vi "Main.vi"(8 "error in":errorcluster, 11 "UI SmarAct in":refnum<class "UI SmarAct.lvclass">) -> (0 "error out":errorcluster, 3 "UI SmarAct out":refnum<class "UI SmarAct.lvclass">)   [LabVIEW 2024, in "UI SmarAct.lvclass"]
doc: "The <b>Queued Message Handler</b> of the Worker that owns this VI."
uses:
  UI SmarAct.lvclass
  C:/Program Files (x86)/National Instruments/LabVIEW 2024/vi.lib/addons/_Workers/Library/Classes/Worker/Worker.lvclass
  <vilib>/addons/_Workers/Library/Classes/Message Queue/Message Queue.lvclass
  <vilib>/addons/_Workers/Library/Classes/Error Handler/Error Handler.lvclass
  <vilib>/addons/_Workers/Library/Classes/Message/Message.lvclass
  <vilib>/addons/_Workers/Library/Classes/EHL/EHL.lvclass
  <vilib>/addons/_Workers/Library/Classes/Workers Object/Workers Object.lvclass
  Spectro Acquisition/Spectro Acquisition.lvclass
  File manipulate/File manipulate.lvclass
  Initialization Data.ctl
  Response Cases.ctl
  UI SmarAct.lvclass/UI SmarAct.ctl
  rql_Connect MCS.ctl
  rql_Update channel.ctl
  rql_Update Vitesse.ctl
  rql_Switch Platine.ctl
  rql_Update Port COM.ctl
  rql_Update Tps Int.ctl
  Spectro Acquisition/rqp_Appliquer BKG.ctl
  rql_Update Calib.ctl
  rql_Update Incr Scan.ctl
  rql_Update fin scan.ctl
  rql_Save Spectrogramme.ctl
  rql_Update Pas Platine.ctl
  rql_Update Controller Adress SMC100.ctl
  Status Platine.ctl
  rql_Refresh.ctl
  rql_Write init file.ctl
  rql_Get position.ctl
  rql_Set Zero Position.ctl
  rql_Find Reference Zero.ctl
  rql_Forward CloseLoop.ctl
  rql_Stop platine.ctl
  rql_Status Position Platine.ctl
  Spectro Acquisition/rqp_Set Int Time.ctl
  rql_Start Acquisition.ctl
  Spectro Acquisition/rqp_Start Acquisition.ctl
  rql_Start Scan.ctl
  File manipulate/rqp_Save Spectrogramme Data.ctl
  Spectro Acquisition/rqp_Appliquer calibration.ctl
  fed1715e-ad66-47da-94cb-5b802a3bcd4b.vi
  338c79d3-4f60-42bd-8753-b5f43bf2242e.vi
  b1e2cd65-b1f1-482f-a644-3403d26b6092.vi
  193bb31d-fb75-400f-a6aa-d82127e562de.vi
  cd9d0536-fc44-4fa3-b225-ca8b7675d591.vi
  9cd4564f-d818-4b39-8ead-d47f8c0a47b5.vi
  <vilib>/ErrorRing/Error Ring.xnode
  <vilib>/addons/_Workers/Debugger/Debug Client/Debug Client.lvlib
panel:
  in  "Commande onglets":T1(tab)
  out "Status Platine":bool
  in  "Platine Newport":enum32{"Initialisation", "Commandes"}(tab)
  in  "Port COM":refnum<visa-resource-name>
  in  "Adresse SMC100":i32
  out "Version Controller":string
  in  "Inc Scan:(um)":dbl step=0.001 format="%#_6f"
  out "fs 3":ext caption="fs" format="%.2f fs"
  out "fs2":ext caption="fs" format="%.2f fs"
  in  "Stop Scan":bool
  in  "fin (um)":i32
  in  "Début (um)":i32
  in  "Start Scan":bool
  out "scan en cours(N)":i32
  in  "Calib?":bool caption="Checkbox"
  in  "BKG":bool
  in  "Stop Acquisition":bool
  in  "Start Acquisition":bool
  in  "Tps Int.(ms)":u32
  out "Connect Spectro?":bool
  in  "Connecter Spectro":bool
  out "Spectrometer Name":string
  out "Serial Number":string
  in  "BKG?":bool caption="Checkbox"
  in  "Platine Switch":bool
  out "Modèle platine":string
  out "fs":ext format="%.2f"
  in  "speed (0 ... 100 000 000)":u32=1000000 max=100000000 step=1
  in  "Channel":u32
  in  "get position":bool
  out "um":dbl format="%.2f"
  in  "Set Zero":bool
  in  "Find Zero":bool
  in  "max freq (50 ... 18 500)":u32=200 min=50 max=18500 step=1
  in  "Stop moteur":bool
  in  "Abs/Rel":bool caption="Checkbox"
  in  "Back CL":bool
  in  "Forward CL":bool
  in  "Inc:(um)":dbl step=0.001 format="%#_6f"
  out "Connect?":bool
  in  "Connecter":bool
  in  "Select MCS":u16(ring)
  in  "Refresh":bool
  out "FWHM(Gauss)":dbl
  out "FWHM(Sech2)":dbl
  out "Aire":dbl
  out "Transposer Le spectrogramme":bool
  in  "Save FROG Trace":bool
  out "Zoom Spectre":cluster{dbl[], dbl[]}(graph)
  out "PosX.Curs-1":dbl
  out "PosX.Curs-0":dbl
  out "Spectre":T2(graph)
  out "Autoccorrélation":dbl[][](graph)
  out "FROG Trace":dbl[][](graph)
  # "Commande Platine Newport"
  # "Scan Platine-Spectro"
  # "Commande Spectromètre"
  # "Modèle Platine :"
  # "Commande Platine MCS"
  # "Commande Platine Closed-Loop"
  # "Connection MCS"
  # "Autoccorrélation"
  # "Reconstruction"
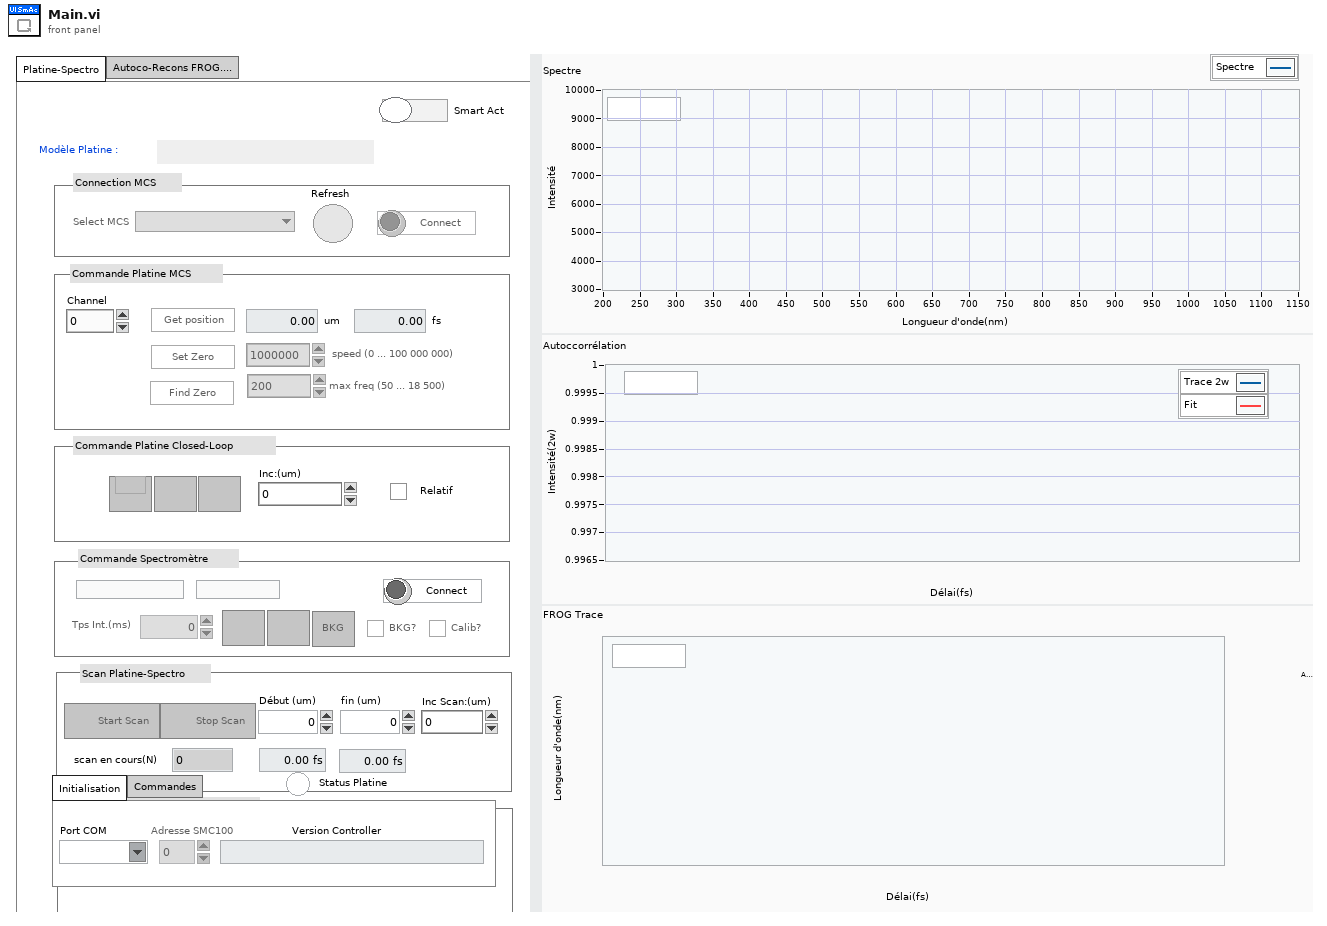
[diagram p1: front panel]
types:
  T1 = enum32{"Platine-Spectro", "Autoco-Recons FROG...."}
  T2 = cluster{"Spectre-BKG":dbl[], "Wavelenghts":dbl[]}
  T3 = cluster{"Wavelenghts":dbl[], "Spectre-BKG":dbl[]}
  T4 = typedef "UI SmarAct.lvclass/Initialization Data.ctl" = cluster{"Response Cases":T5}
  T5 = typedef "UI SmarAct.lvclass/Response Cases.ctl" = cluster{"Placeholder - Can be deleted":string, "Channel":u32, "chemin fichier init":path, "max freq (50 ... 18 500)":u32, "speed (0 ... 100 000 000)":u32, "Abs/Rel":bool, "Tps Int(ms)":u32, "Modèle Platine":string, "Début (um)":i32, "fin (um)":i32, "Inc:(um)":dbl, "Platine Switch":bool, "Port COM":refnum<visa-resource-name>, "Calib?":bool, "Inc Scan:(um)":dbl, "Adresse SMC100":i32}
  T6 = typedef "UI SmarAct.lvclass/Status Platine.ctl" = enum16{"En mouvement...", "Stopée", "Veille"}
  T7 = typedef "UI SmarAct.lvclass/rql_Connect MCS.ctl" = cluster{"String":string, "Connect?":bool}
  T8 = typedef "UI SmarAct.lvclass/rql_Refresh.ctl" = cluster{"String":string}
  T9 = typedef "UI SmarAct.lvclass/rql_Write init file.ctl" = cluster{"String":string}
  T10 = typedef "UI SmarAct.lvclass/rql_Update channel.ctl" = cluster{"Channel":u32}
  T11 = enum32{"SA_SENSOR_DISABLED", "SA_SENSOR_ENABLED", "SA_SENSOR_POWERSAVE"}
  T12 = typedef "UI SmarAct.lvclass/rql_Get position.ctl" = cluster{"String":string}
  T13 = typedef "UI SmarAct.lvclass/rql_Set Zero Position.ctl" = cluster{"String":string}
  T14 = enum32{"SA_FORWARD_DIRECTION", "SA_BACKWARD_DIRECTION", "SA_FORWARD_BACKWARD_DIRECTION", "SA_BACKWARD_FORWARD_DIRECTION", "SA_FORWARD_DIRECTION_ABORT_ON_ENDSTOP", "SA_BACKWARD_DIRECTION_ABORT_ON_ENDSTOP", "SA_FORWARD_BACKWARD_DIRECTION_ABORT_ON_ENDSTOP", "SA_BACKWARD_FORWARD_DIRECTION_ABORT_ON_ENDSTOP"}
  T15 = typedef "UI SmarAct.lvclass/rql_Find Reference Zero.ctl" = cluster{"String":string}
  T16 = typedef "UI SmarAct.lvclass/rql_Forward CloseLoop.ctl" = cluster{"String":string}
  T17 = typedef "UI SmarAct.lvclass/rql_Update Fréquence.ctl" = cluster{"max freq (50 ... 18 500)":u32}
  T18 = typedef "UI SmarAct.lvclass/rql_Update Vitesse.ctl" = cluster{"speed (0 ... 100 000 000)":u32}
  T19 = typedef "UI SmarAct.lvclass/rql_Mode déplacement.ctl" = cluster{"Abs/Rel":bool}
  T20 = typedef "UI SmarAct.lvclass/rql_Initialise Spectromètre.ctl" = cluster{"Connecter Spectro?":bool}
  T21 = typedef "UI SmarAct.lvclass/rql_Stop platine.ctl" = cluster{"String":string}
  T22 = typedef "UI SmarAct.lvclass/rql_Status Position Platine.ctl" = cluster{"String":string}
  T23 = typedef "Spectro Acquisition.lvclass/rqp_Set Int Time.ctl" = cluster{"Tps Int(ms)":u32}
  T24 = typedef "UI SmarAct.lvclass/rql_Update Tps Int.ctl" = cluster{"Tps Int.(ms)":u32}
  T25 = typedef "Spectro Acquisition.lvclass/rqp_Start Acquisition.ctl" = cluster{"Wrapper Spectro":u32}
  T26 = typedef "UI SmarAct.lvclass/rql_Start Acquisition.ctl" = cluster{"String":string}
  T27 = typedef "UI SmarAct.lvclass/rql_Start Scan.ctl" = cluster{"String":string}
  T28 = typedef "UI SmarAct.lvclass/rql_Update début scan.ctl" = cluster{"Début (um)":i32}
  T29 = typedef "UI SmarAct.lvclass/rql_Update fin scan.ctl" = cluster{"fin (um)":i32}
  T30 = typedef "File manipulate.lvclass/rqp_Save Spectrogramme Data.ctl" = cluster{"Save SpecTG":bool, "Paramètres longueur d'onde":T31, "FROG Trace":dbl[][], "pas (um)":dbl, "Nbre de scans":i32, "WL Values":dbl[], "Transposer L'image":bool}
  T31 = typedef "UI SmarAct.lvclass/Paramètres longueur d'onde.ctl" = cluster{"N":i32, "lambda_0":dbl, "lambda_c":dbl, "d_lambda":dbl}
  T32 = typedef "UI SmarAct.lvclass/rql_Save Spectrogramme.ctl" = cluster{"Save":bool}
  T33 = typedef "UI SmarAct.lvclass/rql_Update Pas Platine.ctl" = cluster{"Inc:(um)":dbl}
  T34 = typedef "UI SmarAct.lvclass/rql_Switch Platine.ctl" = cluster{"Platine Switch":bool}
  T35 = typedef "UI SmarAct.lvclass/rql_Update Port COM.ctl" = cluster{"Port COM":refnum<visa-resource-name>}
  T36 = typedef "Spectro Acquisition.lvclass/rqp_Appliquer calibration.ctl" = cluster{"Calib?":bool}
  T37 = typedef "UI SmarAct.lvclass/rql_Update Calib.ctl" = cluster{"Calib?":bool}
  T38 = typedef "UI SmarAct.lvclass/rql_Update Incr Scan.ctl" = cluster{"Inc Scan:(um)":dbl}
  T39 = typedef "UI SmarAct.lvclass/rql_Update Controller Adress SMC100.ctl" = cluster{"Adresse SMC100":i32}
  T40 = typedef "Spectro Acquisition.lvclass/rqp_Appliquer BKG.ctl" = cluster{"BackGround?":bool}
  T41 = enum32{"SA_STOPPED_STATUS", "SA_STEPPING_STATUS", "SA_SCANNING_STATUS", "SA_HOLDING_STATUS", "SA_TARGET_STATUS", "SA_MOVE_DELAY_STATUS", "SA_CALIBRATING_STATUS", "SA_FINDING_REF_STATUS", "SA_OPENING_STATUS"}
  T42 = enum32{"invalid app kind", "Development System", "Run Time System", "Student Edition", "Embedded LabVIEW", "Evaluation", "Custom"}
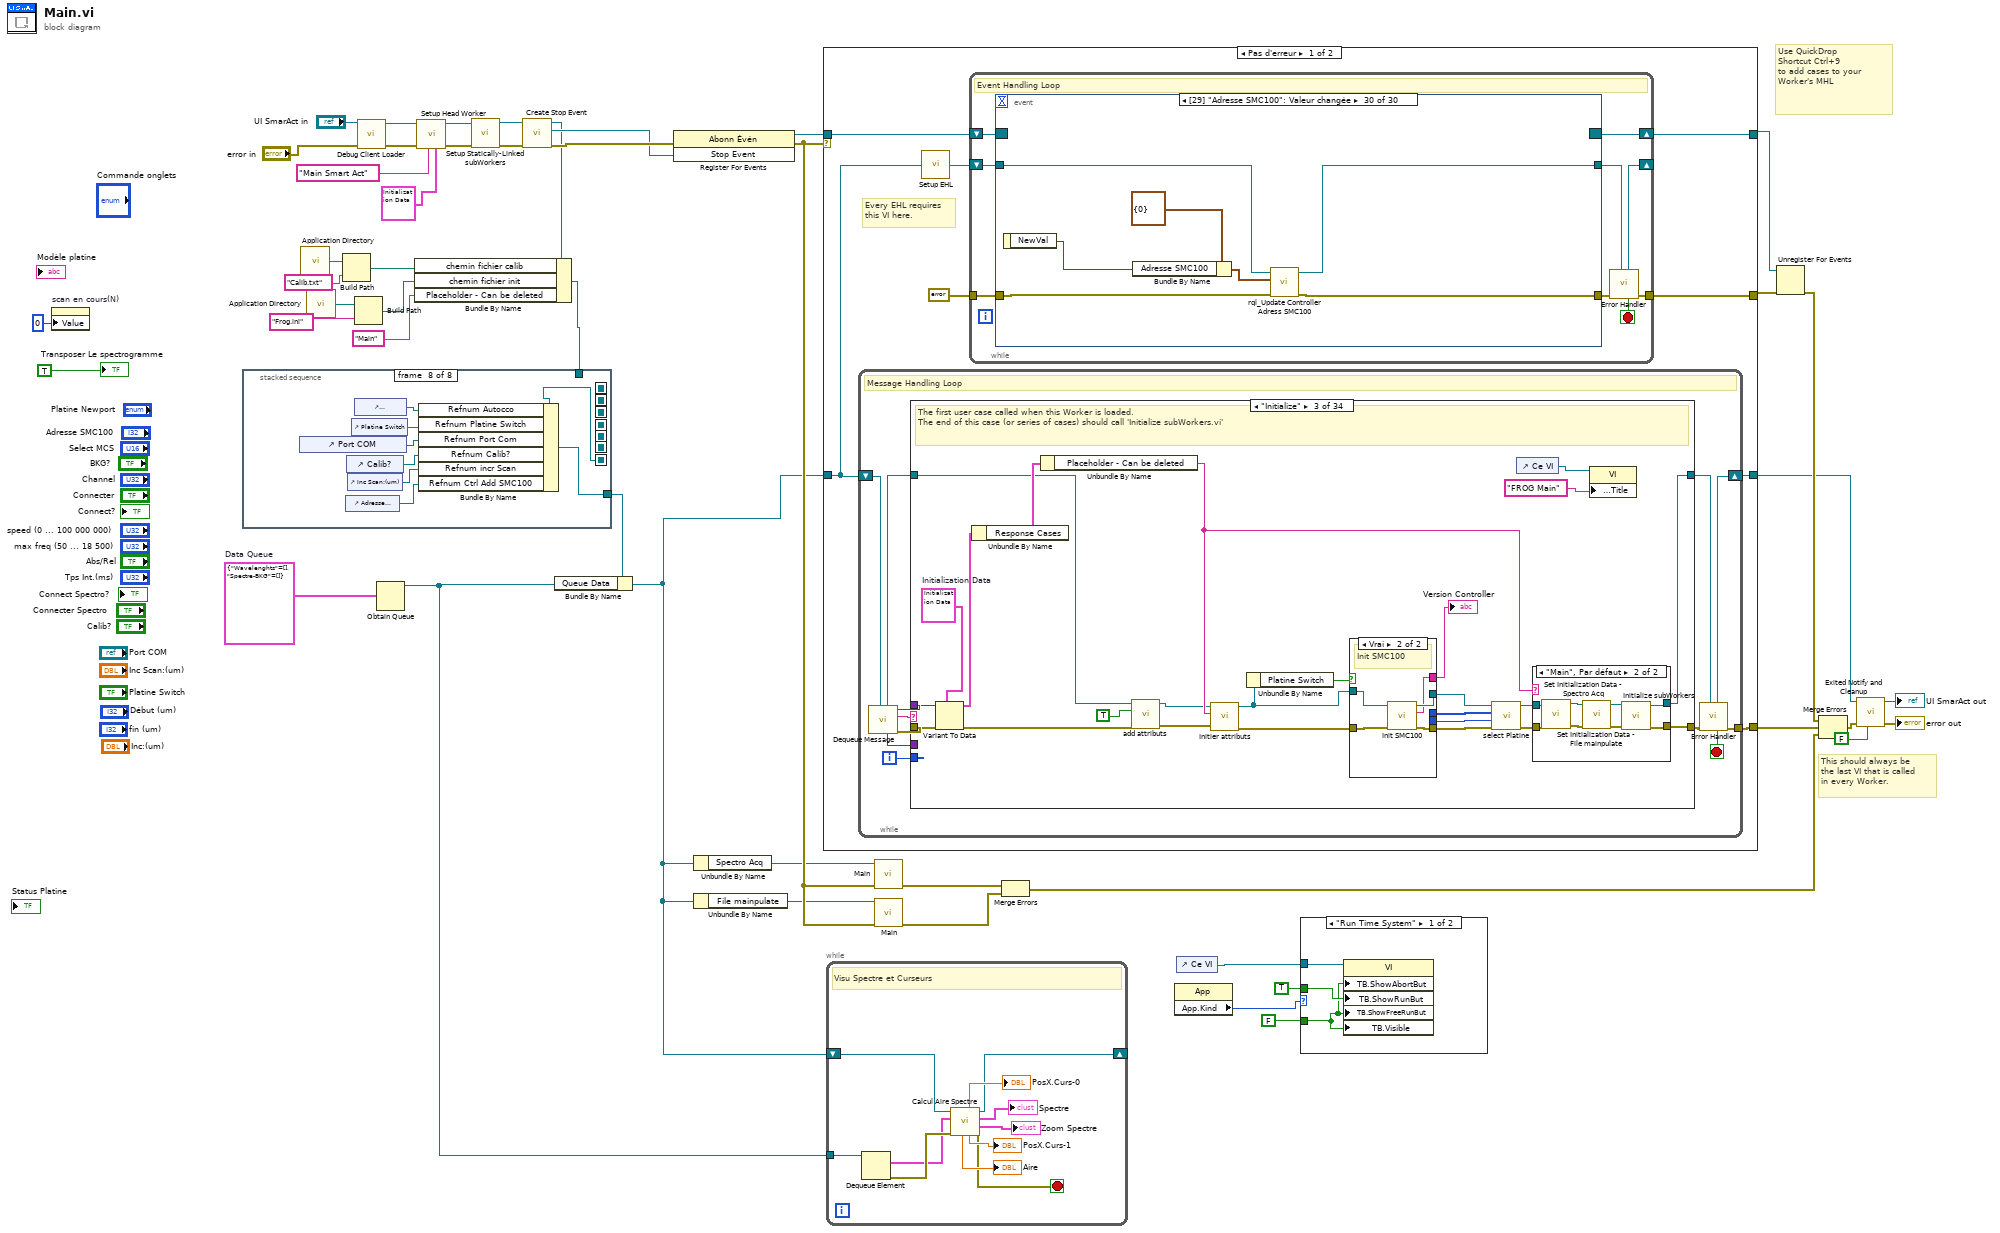
[diagram p0: block diagram]
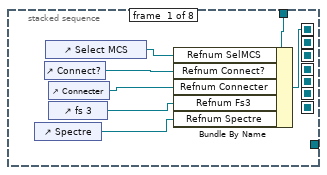
[diagram p2: hidden frame]
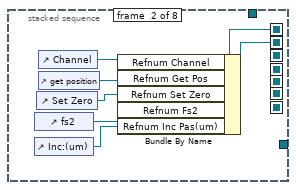
[diagram p3: hidden frame]
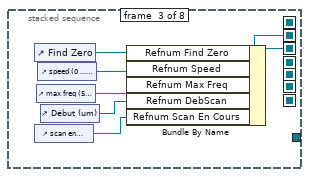
[diagram p4: hidden frame]
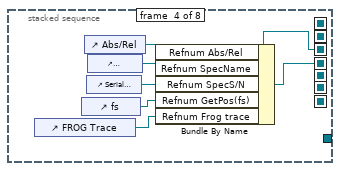
[diagram p5: hidden frame]
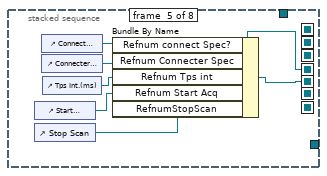
[diagram p6: hidden frame]
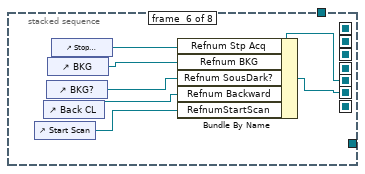
[diagram p7: hidden frame]
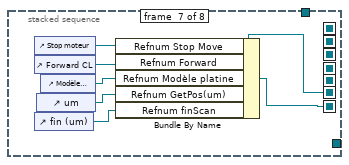
[diagram p8: hidden frame]
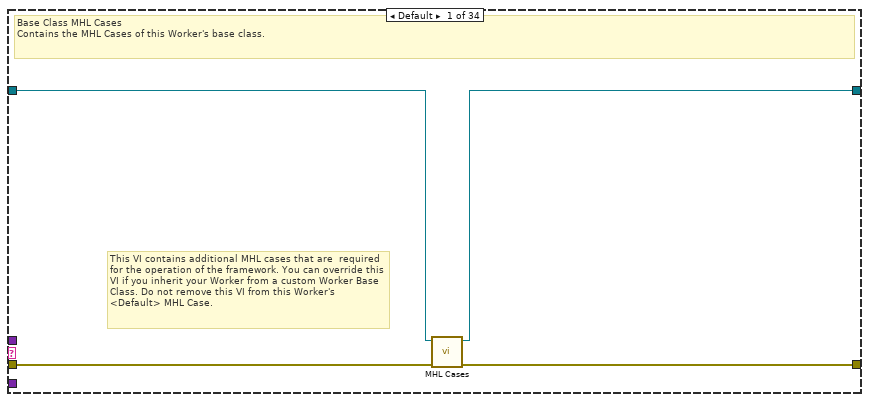
[diagram p10: hidden frame]
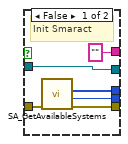
[diagram p12: hidden frame]
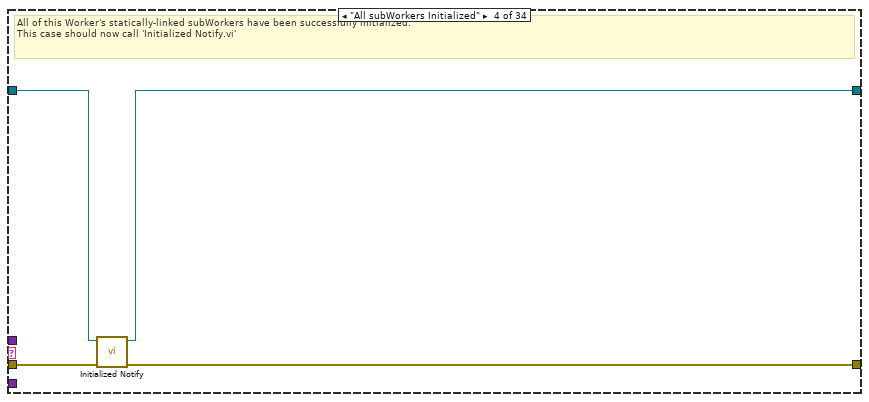
[diagram p14: hidden frame]
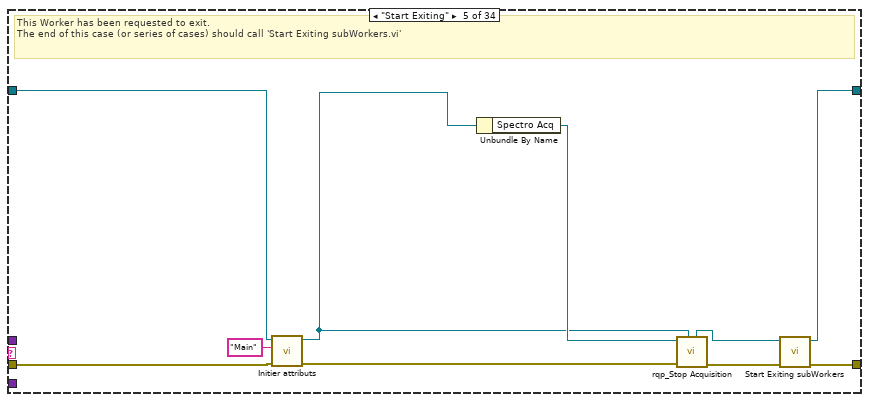
[diagram p15: hidden frame]
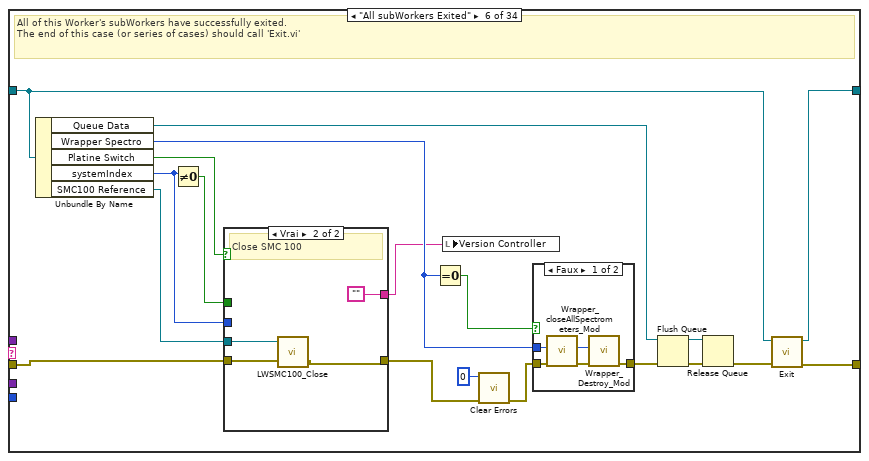
[diagram p16: hidden frame]
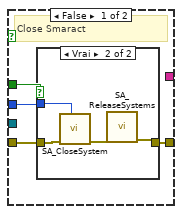
[diagram p17: hidden frame]
diagram:
  w23 = T3 {"Wavelenghts"=[], "Spectre-BKG"=[]}  # Data Queue
  # "Use QuickDrop\nShortcut Ctrl+9\nto add cases to your\nWorker's MHL"
  # "This should always be the last VI that is called in every Worker."
  n1 = property on="scan en cours(N)" class="NumNb (strict)"("Value"=0 ("scan en cours(N)")) -> ()  [unwired: 2 in, 2 out]
  n2 = call <vilib>:"Application Directory.vi"() -> ("Application Directory"=w13:path)
  n3 = call <vilib>:"Application Directory.vi"() -> ("Application Directory"=w33:path)
  n4 = Build Path(base path=w13, name or relative path="Calib.txt") -> (appended path=w7:path)
  n5 = Build Path(base path=w33, name or relative path="Frog.ini") -> (appended path=w6:path)
  n6 = call <vilib>:"Debug Client Loader.vi"("error in (no error)"="error in", "Worker_"="UI SmarAct in") -> ("error out"=w16:errorcluster, "Worker_out"=w15:refnum<class "UI SmarAct.lvclass">)  [unwired: 8 in]
  n7 = Obtain Queue(element data type=w23) -> (queue out=w3:refnum<queue>)  [unwired: 4 in, 2 out]
  n8 = call-dynamic "Setup Head Worker.vi"("Initalization Data"=T4 {"Response Cases"={"Placeholder - Can be deleted"="", "Channel"=0, "chemin fichier init"=path "", "max freq (50 ... 18 500)"=200, "speed (0 ... 100 000 000)"=1000000, "Abs/Rel"=FALSE, "Tps Int(ms)"=0, "Modèle Platine"="", "Début (um)"=0, "fin (um)"=0, "Inc:(um)"=0.0, "Platine Switch"=FALSE, "Port COM"="", "Calib?"=FALSE, "Inc Scan:(um)"=0.0, "Adresse SMC100"=0}} ("Initialization Data"), "Worker Alias"="Main Smart Act", "error in"=w16, "Worker_"=w15) -> ("error out"=w24:errorcluster, "Worker_out"=w27:refnum<class "UI SmarAct.lvclass">)  [unwired: 6 in]
  n9 = call "Setup Statically-Linked subWorkers.vi"("error in"=w24, "UI SmarAct in"=w27) -> ("error out"=w25:errorcluster, "UI SmarAct out"=w26:refnum<class "UI SmarAct.lvclass">)  [unwired: 8 in]
  n10 = call-dynamic "Create Stop Event.vi"("error in"=w25, "Worker"=w26) -> ("error out"=w42:errorcluster, "Stop Event"=w39:refnum<user-event>, "Worker out"=w8:refnum<class "UI SmarAct.lvclass">)  [unwired: 7 in]
  n11 = Bundle By Name ("Assembler par nom")(cluster=w8, "chemin fichier calib"=w7, "chemin fichier init"=w6, "Placeholder - Can be deleted"="Main" ("Response Cases.Placeholder - Can be deleted")) -> (w2:refnum<class "UI SmarAct.lvclass">)
  n12 = stacked-sequence {
    seq-local: [w51 _ _ _ _ _ _ _] -> [_ w61 _ _ _ _ _ _]
    seq-local: [_ w60 _ _ _ _ _ _] -> [_ _ w68 _ _ _ _ _]
    seq-local: [_ _ w64 _ _ _ _ _] -> [_ _ _ w75 _ _ _ _]
    seq-local: [_ _ _ w71 _ _ _ _] -> [_ _ _ _ w78 _ _ _]
    seq-local: [_ _ _ _ w77 _ _ _] -> [_ _ _ _ _ w85 _ _]
    seq-local: [_ _ _ _ _ w84 _ _] -> [_ _ _ _ _ _ w92 _]
    seq-local: [_ _ _ _ _ _ w90 _] -> [_ _ _ _ _ _ _ w98]
    tunnel: w2 -> [w52 _ _ _ _ _ _ _]
    tunnel: [_ _ _ _ _ _ _ w99] -> w1
    frame #0 {
      n13 = control-ref of="Spectre"() -> (w48:refnum<vi>)
      n14 = control-ref of="Connect?"() -> (w53:refnum<vi>)
      n15 = control-ref of="Select MCS"() -> (w54:refnum<vi>)
      n16 = control-ref of="Connecter"() -> (w50:refnum<vi>)
      n17 = control-ref of="fs 3"() -> (w49:refnum<vi>)
      n18 = Bundle By Name ("Assembler par nom")(cluster=w52, "Refnum SelMCS"=w54, "Refnum Connect?"=w53, "Refnum Connecter"=w50, "Refnum Fs3"=w49, "Refnum Spectre"=w48) -> (w51:refnum<class "UI SmarAct.lvclass">)
    }
    frame #1 {
      n19 = control-ref of="fs2"() -> (w56:refnum<vi>)
      n20 = control-ref of="Inc:(um)"() -> (w55:refnum<vi>)
      n21 = control-ref of="Set Zero"() -> (w57:refnum<vi>)
      n22 = control-ref of="Channel"() -> (w59:refnum<vi>)
      n23 = control-ref of="get position"() -> (w58:refnum<vi>)
      n24 = Bundle By Name ("Assembler par nom")(cluster=w61, "Refnum Channel"=w59, "Refnum Get Pos"=w58, "Refnum Set Zero"=w57, "Refnum Fs2"=w56, "Refnum Inc Pas(um)"=w55) -> (w60:refnum<class "UI SmarAct.lvclass">)
    }
    frame #2 {
      n25 = control-ref of="Find Zero"() -> (w65:refnum<vi>)
      n26 = control-ref of="scan en cours(N)"() -> (w62:refnum<vi>)
      n27 = control-ref of="max freq (50 ... 18 500)"() -> (w67:refnum<vi>)
      n28 = control-ref of="speed (0 ... 100 000 000)"() -> (w66:refnum<vi>)
      n29 = control-ref of="Début (um)"() -> (w63:refnum<vi>)
      n30 = Bundle By Name ("Assembler par nom")(cluster=w68, "Refnum Find Zero"=w65, "Refnum Speed"=w66, "Refnum Max Freq"=w67, "Refnum DebScan"=w63, "Refnum Scan En Cours"=w62) -> (w64:refnum<class "UI SmarAct.lvclass">)
    }
    frame #3 {
      n31 = control-ref of="FROG Trace"() -> (w69:refnum<vi>)
      n32 = control-ref of="fs"() -> (w70:refnum<vi>)
      n33 = control-ref of="Abs/Rel"() -> (w74:refnum<vi>)
      n34 = control-ref of="Serial Number"() -> (w72:refnum<vi>)
      n35 = control-ref of="Spectrometer Name"() -> (w73:refnum<vi>)
      n36 = Bundle By Name ("Assembler par nom")(cluster=w75, "Refnum Abs/Rel"=w74, "Refnum SpecName"=w73, "Refnum SpecS/N"=w72, "Refnum GetPos(fs)"=w70, "Refnum Frog trace"=w69) -> (w71:refnum<class "UI SmarAct.lvclass">)
    }
    frame #4 {
      n37 = control-ref of="Start Acquisition"() -> (w79:refnum<vi>)
      n38 = control-ref of="Stop Scan"() -> (w76:refnum<vi>)
      n39 = control-ref of="Connect Spectro?"() -> (w82:refnum<vi>)
      n40 = control-ref of="Connecter Spectro"() -> (w81:refnum<vi>)
      n41 = control-ref of="Tps Int.(ms)"() -> (w80:refnum<vi>)
      n42 = Bundle By Name ("Assembler par nom")(cluster=w78, "Refnum connect Spec?"=w82, "Refnum Connecter Spec"=w81, "Refnum Tps int"=w80, "Refnum Start Acq"=w79, "RefnumStopScan"=w76) -> (w77:refnum<class "UI SmarAct.lvclass">)
    }
    frame #5 {
      n43 = control-ref of="Start Scan"() -> (w83:refnum<vi>)
      n44 = control-ref of="Back CL"() -> (w86:refnum<vi>)
      n45 = control-ref of="BKG?"() -> (w87:refnum<vi>)
      n46 = control-ref of="BKG"() -> (w88:refnum<vi>)
      n47 = control-ref of="Stop Acquisition"() -> (w89:refnum<vi>)
      n48 = Bundle By Name ("Assembler par nom")(cluster=w85, "Refnum Stp Acq"=w89, "Refnum BKG"=w88, "Refnum SousDark?"=w87, "Refnum Backward"=w86, "RefnumStartScan"=w83) -> (w84:refnum<class "UI SmarAct.lvclass">)
    }
    frame #6 {
      n49 = control-ref of="Stop moteur"() -> (w96:refnum<vi>)
      n50 = control-ref of="Forward CL"() -> (w95:refnum<vi>)
      n51 = control-ref of="fin (um)"() -> (w91:refnum<vi>)
      n52 = control-ref of="um"() -> (w93:refnum<vi>)
      n53 = control-ref of="Modèle platine"() -> (w94:refnum<vi>)
      n54 = Bundle By Name ("Assembler par nom")(cluster=w92, "Refnum Stop Move"=w96, "Refnum Forward"=w95, "Refnum Modèle platine"=w94, "Refnum GetPos(um)"=w93, "Refnum finScan"=w91) -> (w90:refnum<class "UI SmarAct.lvclass">)
    }
    frame #7 {
      n55 = control-ref of="Port COM"() -> (w102:refnum<vi>)
      n56 = control-ref of="Adresse SMC100"() -> (w97:refnum<vi>)
      n57 = control-ref of="Calib?"() -> (w101:refnum<vi>)
      n58 = control-ref of="Inc Scan:(um)"() -> (w100:refnum<vi>)
      n59 = control-ref of="Platine Switch"() -> (w103:refnum<vi>)
      n60 = control-ref of="Autoccorrélation"() -> (w104:refnum<vi>)
      n61 = Bundle By Name ("Assembler par nom")(cluster=w98, "Refnum Autocco"=w104, "Refnum Platine Switch"=w103, "Refnum Port Com"=w102, "Refnum Calib?"=w101, "Refnum incr Scan"=w100, "Refnum Ctrl Add SMC100"=w97) -> (w99:refnum<class "UI SmarAct.lvclass">)
    }
  }
  n62 = Bundle By Name ("Assembler par nom")(cluster=w1, "Queue Data"=w3) -> (w4:refnum<class "UI SmarAct.lvclass">)
  n63 = register-events(error in=w42, w39) -> (reference out=w41:refnum<event-registration>, error out=w36:errorcluster)  [unwired: 1 in]
  n64 = Unbundle By Name(w4) -> ("Spectro Acq"=w10:refnum<class "Spectro Acquisition.lvclass">)
  n65 = Unbundle By Name(w4) -> ("File mainpulate"=w9:refnum<class "File manipulate.lvclass">)
  n66 = case shown="Pas d'erreur" w36 {
    tunnel: w4 -> [w107 w942]
    tunnel: [w105 w943] -> w40
    tunnel: w41 -> [w112 w944]
    tunnel: [w109 w945] -> w46
    tunnel: [w111 w944] -> w45
    tunnel: [w106 w941] -> w43
    selector: w36 -> [_ w945]
    frame No Error {
      # "Every EHL requires\nthis VI here."
      n67 = while {
        shift-right: [w122] -> w106
        shift-left: w107 -> [w124]
        tunnel: [w123] -> w105
        i -> [w115]
        stop <- w116 stop-if-true
        # "Message Handling Loop"
        n68 = call-dynamic "Dequeue Message.vi"("Worker"=w124) -> ("error out"=w121:errorcluster, "Case out"=w117:string, "Data out"=w113:variant, "Auxiliary out"=w114:variant, "Worker out"=w119:refnum<class "UI SmarAct.lvclass">)  [unwired: 6 in]
        n69 = case "Worker MHL Case Structure (DO NOT CHANGE LABEL NAME)" shown="\"Initialize\"" w117 {
          tunnel: w121 -> [w128 w129 w155 w178 w187 w206 w230 w247 w270 w279 w288 w312 w324 w336 w354 w402 w442 w453 w464 w478 w492 w505 w551 w563 w574 w639 w652 w672 w682 w696 w710 w728 w740 w753]
          tunnel: [w127 w129 w144 w177 w190 w209 w230 w234 w261 w273 w283 w304 w315 w330 w354 w393 w439 w445 w459 w468 w488 w500 w547 w556 w570 w628 w642 w666 w677 w689 w705 w716 w730 w745] -> w120
          tunnel: w119 -> [w126 w130 w139 w180 w188 w207 w229 w242 w260 w272 w289 w307 w314 w327 w343 w388 w436 w454 w458 w472 w487 w496 w552 w559 w567 w632 w653 w660 w676 w697 w711 w718 w741 w754]
          tunnel: [w125 w130 w143 w179 w189 w208 w229 w233 w265 w271 w281 w307 w313 w327 w345 w385 w438 w443 w457 w465 w486 w498 w546 w559 w569 w626 w645 w664 w675 w688 w704 w714 w732 w743] -> w118
          tunnel: w115 -> [_ _ _ _ _ _ _ _ _ _ _ _ _ _ _ _ _ _ _ _ _ _ _ _ _ _ _ _ _ _ _ _ _ _]
          tunnel: w114 -> [_ _ _ _ _ _ _ _ _ _ _ _ _ _ _ _ _ _ _ _ _ _ _ _ _ _ _ _ _ _ _ _ _ _]
          tunnel: w113 -> [_ _ w154 _ _ _ _ w245 w268 w277 w286 w310 w322 w334 w352 w399 w440 w451 w462 w476 w490 w503 w549 w561 w572 w637 w650 w670 w680 w693 w708 w725 w737 w750]
          frame Default {
            # "This VI contains additional MHL cases that are  required for the operation of the framework. You can override this VI if you inherit your Worker from a custom Worker Base Class. Do not remove this VI from this Worker's <Default> MHL Case."
            # "Base Class MHL Cases\nContains the MHL Cases of this Worker's base class."
            n70 = call-dynamic "MHL Cases.vi"("error in"=w128, "Worker in"=w126) -> ("error out"=w127:errorcluster, "Worker out"=w125:refnum<class "UI SmarAct.lvclass">)  [unwired: 8 in]
          }
          frame "------------ FRAMEWORK CASES -----------" {
            # "Start of Workers Framework Cases"
          }
          frame "Initialize" {
            w153 = T4 {"Response Cases"={"Placeholder - Can be deleted"="", "Channel"=0, "chemin fichier init"=path "", "max freq (50 ... 18 500)"=200, "speed (0 ... 100 000 000)"=1000000, "Abs/Rel"=FALSE, "Tps Int(ms)"=0, "Modèle Platine"="", "Début (um)"=0, "fin (um)"=0, "Inc:(um)"=0.0, "Platine Switch"=FALSE, "Port COM"="", "Calib?"=FALSE, "Inc Scan:(um)"=0.0, "Adresse SMC100"=0}}  # Initialization Data
            # "The first user case called when this Worker is loaded.\nThe end of this case (or series of cases) should call 'Initialize subWorkers.vi'"
            n71 = Variant To Data(error in=w155, type=w153, Variant=w154) -> (data=w148:T4, error out=w137:errorcluster)
            n72 = Unbundle By Name(w148) -> ("Response Cases"=w147:T5)
            n73 = Unbundle By Name(w147) -> ("Placeholder - Can be deleted"=w142:string)
            n74 = call "add attributs.vi"("error in (no error)"=w137, "Read/Write"=TRUE, "UI SA en entrée"=w139) -> ("error out"=w136:errorcluster, "UI SA en sortie"=w138:refnum<class "UI SmarAct.lvclass">)  [unwired: 7 in]
            n75 = call "Initier attributs.vi"("error in (no error)"=w136, "Main/Refresh"=w142, "UI SA en entrée"=w138) -> ("error out"=w149:errorcluster, "UI SA en sortie"=w133:refnum<class "UI SmarAct.lvclass">)  [unwired: 7 in]
            n76 = Unbundle By Name(w133) -> ("Platine Switch"=w134:bool)
            n77 = case shown="Vrai" w134 {
              tunnel: [w161 _] -> w152
              tunnel: [w160 _] -> w151
              tunnel: [w159 w165] -> w150
              tunnel: w149 -> [w158 w166]
              tunnel: w133 -> [w157 w163]
              tunnel: [w157 w164] -> w132
              tunnel: ["" ("ControllerVersion") w162] -> w131
              frame False {
                # "Init Smaract"
                n78 = call <vilib>:"SA_GetAvailableSystems.vi"("error in (no error)"=w158) -> ("error out"=w159:errorcluster, "idListSize out"=w161:u32, "idList"=w160:u32[])  [unwired: 8 in]
              }
              frame True {
                # "Init SMC100"
                n79 = call "Init SMC100.vi"("error in (no error)"=w166, "UI SA en entrée"=w163) -> ("error out"=w165:errorcluster, "ControllerVersion"=w162:string, "UI SA en sortie"=w164:refnum<class "UI SmarAct.lvclass">)  [unwired: 6 in, 1 out]
              }
            }
            "Version Controller" <- w131
            n80 = call "select Platine.vi"("error in"=w150, "idListSize"=w152, "idList"=w151, "UI SmarAct in"=w132) -> ("error out"=w145:errorcluster, "UI SmarAct out"=w146:refnum<class "UI SmarAct.lvclass">)  [unwired: 6 in]
            n81 = control-ref of="Ce VI"() -> (w141:refnum<vi>)
            n82 = case shown="\"Main\", Par défaut" w142 {
              tunnel: w146 -> [w168 w176]
              tunnel: w145 -> [w167 w175]
              tunnel: [w167 w174] -> w144
              tunnel: [w168 w173] -> w143
              frame "Refresh" {
              }
              frame "Main", Default {
                n83 = call "Set Initialization Data - Spectro Acq.vi"("error in"=w175, "UI SmarAct in"=w176) -> ("error out"=w172:errorcluster, "UI SmarAct out"=w170:refnum<class "UI SmarAct.lvclass">)  [unwired: 8 in]
                n84 = call "Set Initialization Data - File mainpulate.vi"("error in"=w172, "UI SmarAct in"=w170) -> ("error out"=w171:errorcluster, "UI SmarAct out"=w169:refnum<class "UI SmarAct.lvclass">)  [unwired: 8 in]
                n85 = call-dynamic "Initialize subWorkers.vi"("error in"=w171, "Worker"=w169) -> ("error out"=w174:errorcluster, "dup Worker out"=w173:refnum<class "UI SmarAct.lvclass">)  [unwired: 8 in]
              }
            }
            n86 = property class="VI"(reference=w141, "Front Panel.Title"="FROG Main" ("Fenêtre face-avant:Titre")) -> ()  [unwired: 1 in, 2 out]
          }
          frame "All subWorkers Initialized" {
            # "All of this Worker's statically-linked subWorkers have been successfully initialized.\nThis case should now call 'Initialized Notify.vi'"
            n87 = call-dynamic "Initialized Notify.vi"("error in"=w178, "Worker"=w180) -> ("error out"=w177:errorcluster, "dup Worker out"=w179:refnum<class "UI SmarAct.lvclass">)  [unwired: 8 in]
          }
          frame "Start Exiting" {
            # "This Worker has been requested to exit. \nThe end of this case (or series of cases) should call 'Start Exiting subWorkers.vi'"
            n88 = call "Initier attributs.vi"("error in (no error)"=w187, "Main/Refresh"="Main", "UI SA en entrée"=w188) -> ("error out"=w186:errorcluster, "UI SA en sortie"=w183:refnum<class "UI SmarAct.lvclass">)  [unwired: 7 in]
            n89 = Unbundle By Name(w183) -> ("Spectro Acq"=w184:refnum<class "Spectro Acquisition.lvclass">)
            n90 = call "rqp_Stop Acquisition.vi"("Caller in"=w183, "error in"=w186, "Spectro Acquisition in"=w184) -> ("error out"=w185:errorcluster, "dup Caller out"=w182:refnum<class "UI SmarAct.lvclass">)  [unwired: 6 in, 1 out]
            n91 = call-dynamic "Start Exiting subWorkers.vi"("error_in"=w185, "Worker"=w182) -> ("error out"=w190:errorcluster, "dup Worker out"=w189:refnum<class "UI SmarAct.lvclass">)  [unwired: 8 in]
          }
          frame "All subWorkers Exited" {
            # "All of this Worker's subWorkers have successfully exited. \nThe end of this case (or series of cases) should call 'Exit.vi'"
            n92 = Unbundle By Name(w207) -> ("Queue Data"=w196:refnum<queue>, "Wrapper Spectro"=w203:u32, "Platine Switch"=w193:bool, "systemIndex"=w204:u32, "SMC100 Reference"=w192:refnum<k24>)
            n93 = Not Equal To 0?(x=w204) -> (x != 0?=w205:bool)
            n94 = case shown="Vrai" w193 {
              tunnel: w206 -> [w213 w222]
              tunnel: w205 -> [w212 _]
              tunnel: w204 -> [w211 _]
              tunnel: [w210 w221] -> w194
              tunnel: w192 -> [_ w220]
              tunnel: [_ ""] -> w191
              frame False {
                # "Close Smaract"
                n95 = case shown="Vrai" w212 {
                  tunnel: w213 -> [w214 w218]
                  tunnel: [w214 w215] -> w210
                  tunnel: w211 -> [_ w217]
                  frame False {
                  }
                  frame True {
                    n96 = call <vilib>:"SA_CloseSystem.vi"("systemIndex"=w217, "error in (no error)"=w218) -> ("error out"=w216:errorcluster)  [unwired: 9 in]
                    n97 = call <vilib>:"SA_ReleaseSystems.vi"("error in (no error)"=w216) -> ("error out"=w215:errorcluster)  [unwired: 10 in]
                  }
                }
              }
              frame True {
                # "Close SMC 100"
                n98 = call "LWSMC100_Close.vi"("error in (no error)"=w222, "CommandInterfaceSMC100.SMC100"=w220) -> ("Error out"=w221:errorcluster)  [unwired: 1 in, 1 out]
              }
            }
            n99 = Equal To 0?(x=w203) -> (x = 0?=w202:bool)
            n100 = local write "Version Controller"(w191) -> ()
            n101 = call <vilib>:"Clear Errors.vi"("error in (no error)"=w194, "specific error code to clear (0: all)"=0) -> ("error out"=w201:errorcluster)  [unwired: 4 in, 1 out]
            n102 = case shown="Faux" w202 {
              tunnel: w201 -> [w227 w228]
              tunnel: w203 -> [w225 _]
              tunnel: [w223 w228] -> w199
              frame False {
                n103 = call "Wrapper_closeAllSpectrometers_Mod.vi"("error in (no error)"=w227, "Wrapper In"=w225) -> ("error out"=w224:errorcluster, "Wrapper Out"=w226:u32)  [unwired: 8 in]
                n104 = call "Wrapper_Destroy_Mod.vi"("error in (no error)"=w224, "Wrapper"=w226) -> ("error out"=w223:errorcluster)  [unwired: 9 in]
              }
              frame True {
              }
            }
            n105 = Flush Queue(queue=w196, error in (no error)=w199) -> (queue out=w195:refnum<queue>, error out=w197:errorcluster)  [unwired: 1 out]
            n106 = Release Queue(queue=w195, error in (no error)=w197) -> (error out=w198:errorcluster)  [unwired: 1 in, 2 out]
            n107 = call-dynamic "Exit.vi"("error_in"=w198, "Worker"=w207) -> ("error out"=w209:errorcluster, "dup Worker out"=w208:refnum<class "UI SmarAct.lvclass">)  [unwired: 8 in]
          }
          frame "------------- LOCAL API CASES -------------" {
            # "Start of Workers Local API Cases"
          }
          frame "Connect MCS" {
            # "Connect MCS"
            n108 = Variant To Data(error in=w247, type=T7 {"String"="", "Connect?"=FALSE} ("Data"), Variant=w245) -> (data=w244:T7, error out=w239:errorcluster)
            n109 = Unbundle By Name(w242) -> ("systemIndex"=w237:u32, "Refnum SelMCS"=w241:refnum<vi>)
            n110 = Unbundle By Name(w244) -> ("Connect?"=w243:bool)
            n111 = property class="MDér (strict)"(reference=w241, error in=w239) -> (error out=w238:errorcluster, "RingText.Text"=w240:string)  [unwired: 1 out]
            n112 = case shown="Faux" w243 {
              tunnel: w240 -> [_ w256]
              tunnel: [u32 0 ("systemIndexOut") w252] -> w236
              tunnel: w237 -> [w251 _]
              tunnel: w238 -> [w250 w255]
              tunnel: [w249 w253] -> w235
              frame False {
                n113 = call <vilib>:"SA_CloseSystem.vi"("systemIndex"=w251, "error in (no error)"=w250) -> ("error out"=w249:errorcluster)  [unwired: 9 in]
              }
              frame True {
                n114 = call <vilib>:"SA_OpenSystem.vi"("error in (no error)"=w255, "options"="sync", "systemLocator"=w256) -> ("error out"=w253:errorcluster, "systemIndexOut"=w252:u32)  [unwired: 7 in]
              }
            }
            n115 = Bundle By Name ("Assembler par nom")(cluster=w242, "systemIndex"=w236, "Status Platine"=Status_Platine."Veille") -> (w232:refnum<class "UI SmarAct.lvclass">)
            n116 = call "MCS connecté.vi"("error in (no error)"=w235, "UI SA en entrée"=w232) -> ("error out"=w234:errorcluster, "UI SA en sortie"=w233:refnum<class "UI SmarAct.lvclass">)  [unwired: 8 in]
          }
          frame "Refresh" {
            # "Ré-initialise le controleur MCS"
            n117 = Variant To Data(error in=w270, type=T8 {"String"=""} ("Data"), Variant=w268) -> (data=w267:T8, error out=w266:errorcluster)
            n118 = Unbundle By Name(w267) -> ()  [unwired: 1 out]
            n119 = call-dynamic "Get Queue.vi"("error in (no error)"=w266, "Worker_"=w260) -> ("error out"=w262:errorcluster, "Message Queue"=w264:refnum<class "Message Queue.lvclass">)  [unwired: 7 in, 1 out]
            n120 = Bundle By Name(cluster=T4 {"Response Cases"={"Placeholder - Can be deleted"="", "Channel"=0, "chemin fichier init"=path "", "max freq (50 ... 18 500)"=200, "speed (0 ... 100 000 000)"=1000000, "Abs/Rel"=FALSE, "Tps Int(ms)"=0, "Modèle Platine"="", "Début (um)"=0, "fin (um)"=0, "Inc:(um)"=0.0, "Platine Switch"=FALSE, "Port COM"="", "Calib?"=FALSE, "Inc Scan:(um)"=0.0, "Adresse SMC100"=0}} ("Initialization Data"), "Response Cases.Placeholder - Can be deleted"="Refresh") -> (w258:T4)
            n121 = call-dynamic "Enqueue Standard Message.vi"("Worker"=w260, "Message Queue"=w264, "Case Label"="Initialize", "Data"=w258, "error in (no error)"=w262) -> ("dup Worker out"=w265:refnum<class "UI SmarAct.lvclass">, "error out"=w261:errorcluster)  [unwired: 9 in]
          }
          frame "Write init file" {
            # "Enregistrer dans le fichier INI"
            n122 = Variant To Data(error in=w279, type=T9 {"String"=""} ("Data"), Variant=w277) -> (data=w276:T9, error out=w274:errorcluster)
            n123 = Unbundle By Name(w276) -> ()  [unwired: 1 out]
            n124 = call "add attributs.vi"("error in (no error)"=w274, "Read/Write"=FALSE, "UI SA en entrée"=w272) -> ("error out"=w273:errorcluster, "UI SA en sortie"=w271:refnum<class "UI SmarAct.lvclass">)  [unwired: 7 in]
          }
          frame "Update channel" {
            # "Modifie la valeur du channel"
            n125 = Variant To Data(error in=w288, type=T10 {"Channel"=0} ("Data"), Variant=w286) -> (data=w285:T10, error out=w284:errorcluster)
            n126 = Unbundle By Name(w285) -> ("Channel"=w280:u32)
            n127 = Bundle By Name ("Assembler par nom")(cluster=w289, "Channel"=w280) -> (w282:refnum<class "UI SmarAct.lvclass">)
            n128 = call "rql_Write init file.vi"("error in"=w284, "UI SmarAct in"=w282) -> ("error out"=w283:errorcluster, "dup UI SmarAct out"=w281:refnum<class "UI SmarAct.lvclass">)  [unwired: 8 in]
          }
          frame "Get position" {
            # "Returns the current position of a positioner. This function is only executable by a positioner that has a sensor\nattached to it. The sensor must also be enabled or in power save mode (see SA_SetSensorEnabled_S)."
            n129 = Variant To Data(error in=w312, type=T12 {"String"=""} ("Data"), Variant=w310) -> (data=w309:T12, error out=w306:errorcluster)
            n130 = Unbundle By Name(w309) -> ()  [unwired: 1 out]
            n131 = Unbundle By Name(w307) -> ("Channel"=w302:u32, "systemIndex"=w303:u32)
            n132 = call <vilib>:"SA_SetSensorEnabled_S.vi"("systemIndex"=w303, "error in (no error)"=w306, "enabled"=T11."SA_SENSOR_ENABLED") -> ("error out"=w305:errorcluster)  [unwired: 8 in]
            n133 = call <vilib>:"SA_GetPosition_S.vi"("channelIndex"=w302, "systemIndex"=w303, "error in (no error)"=w305) -> ("error out"=w304:errorcluster, "position"=w301:i32)  [unwired: 7 in]
            n134 = To Double Precision Float(number=w301) -> (double precision float=w299:dbl)
            n135 = Divide(x=w299, y=1000.0) -> (x/y=w295:dbl)
            "um" <- w295
            n136 = Multiply(x=w295, y=1e-06) -> (x*y=w293:dbl)
            n137 = Divide(x=w293, y=ext[unit] 300000000.0) -> (x/y=w298:ext[unit])
            n138 = Multiply(x=w298, y=ext[unit] 1000000000000000.0) -> (x*y=w292:ext)
            n139 = Multiply(x=w292, y=ext 2.0) -> (x*y=→"fs":ext)
          }
          frame "Set Zero Position" {
            # "For positioners that have a sensor installed, this function may be used to define the current position resp.\nangle of the positioner to have a specific value (par ex 0)"
            n140 = Variant To Data(error in=w324, type=T13 {"String"=""} ("Data"), Variant=w322) -> (data=w321:T13, error out=w320:errorcluster)
            n141 = Unbundle By Name(w321) -> ()  [unwired: 1 out]
            n142 = Unbundle By Name(w314) -> ("Channel"=w318:u32, "systemIndex"=w317:u32)
            n143 = call <vilib>:"SA_SetPosition_S.vi"("channelIndex"=w318, "systemIndex"=w317, "error in (no error)"=w320, "position"=0) -> ("error out"=w316:errorcluster)  [unwired: 7 in]
            n144 = call "rql_Get position.vi"("error in"=w316, "UI SmarAct in"=w314) -> ("error out"=w315:errorcluster, "dup UI SmarAct out"=w313:refnum<class "UI SmarAct.lvclass">)  [unwired: 8 in]
          }
          frame "Find Reference Zero" {
            # "For positioners that are equipped with sensor feedback, this function may be used to move the positioner to\na known physical position of the positioner"
            n145 = Variant To Data(error in=w336, type=T15 {"String"=""} ("Data"), Variant=w334) -> (data=w333:T15, error out=w331:errorcluster)
            n146 = Unbundle By Name(w333) -> ()  [unwired: 1 out]
            n147 = Unbundle By Name(w327) -> ("Channel"=w326:u32, "systemIndex"=w325:u32)
            n148 = call <vilib>:"SA_FindReferenceMark_S.vi"("channelIndex"=w326, "systemIndex"=w325, "error in (no error)"=w331, "autoZero"=enum32{"SA_NO_AUTO_ZERO", "SA_AUTO_ZERO"}."SA_NO_AUTO_ZERO", "holdTime"=u32 0, "direction"=T14."SA_FORWARD_DIRECTION") -> ("error out"=w330:errorcluster)  [unwired: 5 in]
          }
          frame "Forward CloseLoop" {
            # "Avance relative en boucle fermée"
            n149 = Unbundle By Name(w343) -> ("Abs/Rel"=w346:bool, "systemIndex"=w340:u32, "Channel"=w339:u32, "Status Platine"=w341:T6, "Inc:(um)"=w338:dbl)
            n150 = Variant To Data(error in=w354, type=T16 {"String"=""} ("Data"), Variant=w352) -> (data=w351:T16, error out=w348:errorcluster)
            n151 = Unbundle By Name(w351) -> ()  [unwired: 1 out]
            n152 = Multiply(x=w338, y=1000.0) -> (x*y=w349:dbl)
            n153 = To Long Integer(number=w349) -> (32bit integer=w337:i32)
            n154 = case shown="\"Veille\"" w341 {
              tunnel: w348 -> [w355 w365 w382]
              tunnel: [w355 w368 w382] -> _
              tunnel: w343 -> [w356 w367 w381]
              tunnel: [w356 w366 w381] -> w342
              tunnel: u32 500 ("holdTime") -> [_ w364 _]
              tunnel: w337 -> [_ w363 _]
              tunnel: w340 -> [_ w362 _]
              tunnel: w339 -> [_ w361 _]
              tunnel: w346 -> [_ w360 _]
              frame "En mouvement...", Default {
              }
              frame "Veille" {
                n155 = case shown="Vrai" w360 {
                  tunnel: [w373 w380] -> w359
                  tunnel: w365 -> [w372 w379]
                  tunnel: w364 -> [w374 w378]
                  tunnel: w363 -> [w371 w377]
                  tunnel: w362 -> [w370 w376]
                  tunnel: w361 -> [w369 w375]
                  frame False {
                    n156 = call <vilib>:"SA_GotoPositionRelative_S.vi"("channelIndex"=w369, "systemIndex"=w370, "error in (no error)"=w372, "holdTime"=w374, "diff"=w371) -> ("error out"=w373:errorcluster)  [unwired: 6 in]
                  }
                  frame True {
                    n157 = call <vilib>:"SA_GotoPositionAbsolute_S.vi"("channelIndex"=w375, "systemIndex"=w376, "error in (no error)"=w379, "holdTime"=w378, "position"=w377) -> ("error out"=w380:errorcluster)  [unwired: 6 in]
                  }
                }
                n158 = call "Stall Data Flow.vim"("value in"=w359, "milliseconds to wait"=u32 100) -> ("value out"=w358:errorcluster)  [unwired: 1 out]
                n159 = call "rql_Status Position Platine.vi"("error in"=w358, "UI SmarAct in"=w367) -> ("error out"=w368:errorcluster, "dup UI SmarAct out"=w366:refnum<class "UI SmarAct.lvclass">)  [unwired: 8 in]
              }
              frame "Stopée" {
              }
            }
            n160 = Bundle By Name ("Assembler par nom")(cluster=w342, "Status Platine"=Status_Platine."En mouvement...") -> (w345:refnum<class "UI SmarAct.lvclass">)
          }
          frame "Back Closed Loog" {
            # "Retour relatif en boucle fermée"
            n161 = Unbundle By Name(w388) -> ("Abs/Rel"=w390:bool, "systemIndex"=w396:u32, "Channel"=w395:u32, "Status Platine"=w389:T6, "Inc:(um)"=w384:dbl)
            n162 = Variant To Data(error in=w402, type=T16 {"String"=""} ("Data"), Variant=w399) -> (data=w400:T16, error out=w394:errorcluster)
            n163 = Unbundle By Name(w400) -> ()  [unwired: 1 out]
            n164 = Multiply(x=w384, y=1000.0) -> (x*y=w398:dbl)
            n165 = Negate(x=w398) -> (-x=w391:dbl)
            n166 = To Long Integer(number=w391) -> (32bit integer=w383:i32)
            n167 = case shown="\"Veille\"" w389 {
              tunnel: u32 500 ("holdTime") -> [_ w416 _]
              tunnel: w396 -> [_ w415 _]
              tunnel: w395 -> [_ w414 _]
              tunnel: w394 -> [w403 w413 w429]
              tunnel: [w403 w410 w429] -> w393
              tunnel: w383 -> [_ w412 _]
              tunnel: w390 -> [_ w411 _]
              tunnel: w388 -> [w404 w409 w430]
              tunnel: [w404 w408 w430] -> w386
              frame "En mouvement...", Default {
              }
              frame "Veille" {
                n168 = case shown="Faux" w411 {
                  tunnel: [w421 w428] -> w406
                  tunnel: w416 -> [w417 w427]
                  tunnel: w415 -> [w420 w426]
                  tunnel: w414 -> [w419 w425]
                  tunnel: w413 -> [w422 w424]
                  tunnel: w412 -> [w418 w423]
                  frame False {
                    n169 = call <vilib>:"SA_GotoPositionRelative_S.vi"("channelIndex"=w419, "systemIndex"=w420, "error in (no error)"=w422, "holdTime"=w417, "diff"=w418) -> ("error out"=w421:errorcluster)  [unwired: 6 in]
                  }
                  frame True {
                    n170 = call <vilib>:"SA_GotoPositionAbsolute_S.vi"("channelIndex"=w425, "systemIndex"=w426, "error in (no error)"=w424, "holdTime"=w427, "position"=w423) -> ("error out"=w428:errorcluster)  [unwired: 6 in]
                  }
                }
                n171 = call "Stall Data Flow.vim"("value in"=w406, "milliseconds to wait"=u32 100) -> ("value out"=w405:errorcluster)  [unwired: 1 out]
                n172 = call "rql_Status Position Platine.vi"("error in"=w405, "UI SmarAct in"=w409) -> ("error out"=w410:errorcluster, "dup UI SmarAct out"=w408:refnum<class "UI SmarAct.lvclass">)  [unwired: 8 in]
              }
              frame "Stopée" {
              }
            }
            n173 = Bundle By Name ("Assembler par nom")(cluster=w386, "Status Platine"=Status_Platine."En mouvement...") -> (w385:refnum<class "UI SmarAct.lvclass">)
          }
          frame "Update Fréquence" {
            # "Mise à jour de la fréquence Max de la platine"
            n174 = Variant To Data(error in=w442, type=T17 {"max freq (50 ... 18 500)"=200} ("Data"), Variant=w440) -> (data=w437:T17, error out=w433:errorcluster)
            n175 = Unbundle By Name(w437) -> ("max freq (50 ... 18 500)"=w431:u32)
            n176 = Bundle By Name ("Assembler par nom")(cluster=w436, "max freq (50 ... 18 500)"=w431) -> (w435:refnum<class "UI SmarAct.lvclass">)
            n177 = call "Set Closed Loop Fréq.vi"("error in (no error)"=w433, "frequency"=w431, "UI SA en entrée"=w435) -> ("error out"=w432:errorcluster, "UI SA en sortie"=w434:refnum<class "UI SmarAct.lvclass">)  [unwired: 7 in]
            n178 = call "rql_Write init file.vi"("error in"=w432, "UI SmarAct in"=w434) -> ("error out"=w439:errorcluster, "dup UI SmarAct out"=w438:refnum<class "UI SmarAct.lvclass">)  [unwired: 8 in]
          }
          frame "Update Vitesse" {
            # "This function configures the speed control feature of a channel for closed-loop commands such as SA_GotoPositionAbsolute_S."
            n179 = Variant To Data(error in=w453, type=T18 {"speed (0 ... 100 000 000)"=1000000} ("Data"), Variant=w451) -> (data=w450:T18, error out=w449:errorcluster)
            n180 = Unbundle By Name(w450) -> ("speed (0 ... 100 000 000)"=w447:u32)
            n181 = Bundle By Name ("Assembler par nom")(cluster=w454, "speed (0 ... 100 000 000)"=w447) -> (w448:refnum<class "UI SmarAct.lvclass">)
            n182 = call "Set Closed Loop Speedvi.vi"("error in (no error)"=w449, "speed"=w447, "UI SA en entrée"=w448) -> ("error out"=w446:errorcluster, "UI SA en sortie"=w444:refnum<class "UI SmarAct.lvclass">)  [unwired: 7 in]
            n183 = call "rql_Write init file.vi"("error in"=w446, "UI SmarAct in"=w444) -> ("error out"=w445:errorcluster, "dup UI SmarAct out"=w443:refnum<class "UI SmarAct.lvclass">)  [unwired: 8 in]
          }
          frame "Mode déplacement" {
            # "Update du mode de éplacement de la platine"
            n184 = Variant To Data(error in=w464, type=T19 {"Abs/Rel"=FALSE} ("Data"), Variant=w462) -> (data=w461:T19, error out=w460:errorcluster)
            n185 = Unbundle By Name(w461) -> ("Abs/Rel"=w455:bool)
            n186 = Bundle By Name ("Assembler par nom")(cluster=w458, "Abs/Rel"=w455) -> (w456:refnum<class "UI SmarAct.lvclass">)
            n187 = call "rql_Write init file.vi"("error in"=w460, "UI SmarAct in"=w456) -> ("error out"=w459:errorcluster, "dup UI SmarAct out"=w457:refnum<class "UI SmarAct.lvclass">)  [unwired: 8 in]
          }
          frame "Initialise Spectromètre" {
            # "Initialisation du spectromètre"
            n188 = Variant To Data(error in=w478, type=T20 {"Connecter Spectro?"=FALSE} ("Data"), Variant=w476) -> (error out=w475:errorcluster)  [unwired: 1 out]
            n189 = Unbundle By Name(w472) -> ("Refnum Connecter Spec"=w471:refnum<vi>)
            n190 = property class="Bool (strict)"(reference=w471) -> ("Value"=w470:bool)  [unwired: 1 in, 2 out]
            n191 = call "Initialisation Spectro.vi"("error in (no error)"=w475, "Connecter?"=w470, "UI SA en entrée"=w472) -> ("error out"=w469:errorcluster, "Serial Number"=→"Serial Number":string, "Spectrometer Name"=→"Spectrometer Name":string, "UI SA en sortie"=w466:refnum<class "UI SmarAct.lvclass">, "Spectro Connecté?"=w467:bool)  [unwired: 4 in]
            n192 = case shown="Vrai" w467 {
              tunnel: w466 -> [w479 w484]
              tunnel: [w479 w483] -> w465
              tunnel: w469 -> [w480 w482]
              tunnel: [w480 w481] -> w468
              frame False {
              }
              frame True {
                n193 = call "Set Tps Int.vi"("error in (no error)"=w482, "UI SA en entrée"=w484) -> ("error out"=w481:errorcluster, "UI SA en sortie"=w483:refnum<class "UI SmarAct.lvclass">)  [unwired: 8 in]
              }
            }
          }
          frame "Stop platine" {
            # "Arrête la platine en cours de déplacement"
            n194 = Variant To Data(error in=w492, type=T21 {"String"=""} ("Data"), Variant=w490) -> (data=w489:T21, error out=w488:errorcluster)
            n195 = Unbundle By Name(w489) -> ()  [unwired: 1 out]
            n196 = Bundle By Name ("Assembler par nom")(cluster=w487, "Status Platine"=Status_Platine."Stopée") -> (w486:refnum<class "UI SmarAct.lvclass">)
          }
          frame "Status Position Platine" {
            # "renvoi le status et la position de la platine"
            n197 = Variant To Data(error in=w505, type=T22 {"String"=""} ("Data"), Variant=w503) -> (data=w502:T22, error out=w501:errorcluster)
            n198 = Unbundle By Name(w496) -> ("Channel"=w493:u32, "systemIndex"=w494:u32, "Status Platine"=w499:T6)
            n199 = Unbundle By Name(w502) -> ()  [unwired: 1 out]
            n200 = case shown="\"En mouvement...\"" w499 {
              tunnel: w501 -> [w521 w532 w537]
              tunnel: [w527 w531 w537] -> w500
              tunnel: [w517 Status_Platine."Veille" ("Status Platine") Status_Platine."Veille" ("Status Platine")] -> w497
              tunnel: w496 -> [w512 w534 w535]
              tunnel: [w526 w534 w535] -> w495
              tunnel: w494 -> [w516 w530 _]
              tunnel: w493 -> [w515 w529 _]
              frame "En mouvement..." {
                n201 = disable-structure shown="Désactivé" {
                  frame Disabled {
                    n202 = Wait Until Next ms Multiple(millisecond multiple=u32 150 ("n millisecondes")) -> ()  [unwired: 1 out]
                  }
                  frame Enabled {
                  }
                }
                n203 = call <vilib>:"SA_GetStatus_S.vi"("channelIndex"=w515, "systemIndex"=w516, "error in (no error)"=w521) -> ("error out"=w525:errorcluster, "status"=w522:T41)  [unwired: 7 in]
                n204 = Equal To 0?(x=w522) -> (x = 0?=w520:bool)
                n205 = call <vilib>:"SA_GetPosition_S.vi"("channelIndex"=w515, "systemIndex"=w516, "error in (no error)"=w525) -> ("error out"=w508:errorcluster, "position"=w524:i32)  [unwired: 7 in]
                n206 = To Double Precision Float(number=w524) -> (double precision float=w523:dbl)
                n207 = Divide(x=w523, y=1000.0) -> (x/y=w511:dbl)
                n208 = call "Stall Data Flow.vim"("value in"=w508, "milliseconds to wait"=u32 150) -> ("value out"=w507:errorcluster)  [unwired: 1 out]
                n209 = local write "um"(w511) -> ()
                n210 = Select(t=Status_Platine."Veille" ("Status Platine"), s=w520, f=Status_Platine."En mouvement..." ("Status Platine")) -> (s? t:f=w517:T6)
                n211 = call "Conversion umToFs.vi"("error in (no error)"=w507, "um"=w511, "UI SA en entrée"=w512) -> ("error out"=w514:errorcluster, "Fs"=w510:ext, "UI SA en sortie"=w513:refnum<class "UI SmarAct.lvclass">)  [unwired: 6 in]
                n212 = local write "fs"(w510) -> ()
                n213 = call "rql_Status Position Platine.vi"("error in"=w514, "UI SmarAct in"=w513) -> ("error out"=w527:errorcluster, "dup UI SmarAct out"=w526:refnum<class "UI SmarAct.lvclass">)  [unwired: 8 in]
              }
              frame "Stopée" {
                n214 = call <vilib>:"SA_Stop_S.vi"("channelIndex"=w529, "systemIndex"=w530, "error in (no error)"=w532) -> ("error out"=w531:errorcluster)  [unwired: 8 in]
              }
              frame "Veille", Default {
              }
            }
            n215 = Bundle By Name ("Assembler par nom")(cluster=w495, "Status Platine"=w497) -> (w498:refnum<class "UI SmarAct.lvclass">)
          }
          frame "Update Tps Int" {
            # "Update le temps d'intégration"
            n216 = Variant To Data(error in=w551, type=T24 {"Tps Int.(ms)"=0} ("Data"), Variant=w549) -> (data=w548:T24, error out=w545:errorcluster)
            n217 = Unbundle By Name(w548) -> ("Tps Int.(ms)"=w538:u32)
            n218 = Bundle By Name ("Assembler par nom")(cluster=w552, "Tps Int(ms)"=w538) -> (w542:refnum<class "UI SmarAct.lvclass">)
            n219 = Bundle By Name(cluster=T23 {"Tps Int(ms)"=0} ("Data in"), "Tps Int(ms)"=w538) -> (w539:T23)
            n220 = Unbundle By Name(w542) -> ("Spectro Acq"=w541:refnum<class "Spectro Acquisition.lvclass">)
            n221 = call "rqp_Set Int Time.vi"("Caller in"=w542, "error in"=w545, "Data in"=w539, "Spectro Acquisition in"=w541) -> ("error out"=w544:errorcluster, "dup Caller out"=w543:refnum<class "UI SmarAct.lvclass">)  [unwired: 5 in, 1 out]
            n222 = call "rql_Write init file.vi"("error in"=w544, "UI SmarAct in"=w543) -> ("error out"=w547:errorcluster, "dup UI SmarAct out"=w546:refnum<class "UI SmarAct.lvclass">)  [unwired: 8 in]
          }
          frame "Start Acquisition" {
            # "Démarre l'acquisition du spectro"
            n223 = Variant To Data(error in=w563, type=T26 {"String"=""} ("Data"), Variant=w561) -> (data=w560:T26, error out=w557:errorcluster)
            n224 = Unbundle By Name(w560) -> ()  [unwired: 1 out]
            n225 = Unbundle By Name(w559) -> ("Spectro Acq"=w555:refnum<class "Spectro Acquisition.lvclass">, "Wrapper Spectro"=w553:u32)
            n226 = Bundle By Name(cluster=T25 {"Wrapper Spectro"=0} ("Data in"), "Wrapper Spectro"=w553) -> (w554:T25)
            n227 = call "rqp_Start Acquisition.vi"("error in"=w557, "Data in"=w554, "Spectro Acquisition in"=w555) -> ("error out"=w556:errorcluster)  [unwired: 6 in, 2 out]
          }
          frame "Start Scan" {
            # "Démarre le scan"
            n228 = Unbundle By Name(w567) -> ("Status Platine"=w566:T6, "Spectro Acq"=w565:refnum<class "Spectro Acquisition.lvclass">, "Inc Scan:(um)"=w564:dbl)
            n229 = Variant To Data(error in=w574, type=T27 {"String"=""} ("Data"), Variant=w572) -> (data=w571:T27, error out=w568:errorcluster)
            n230 = Unbundle By Name(w571) -> ()  [unwired: 1 out]
            n231 = case shown="\"Veille\"" w566 {
              tunnel: [w575 w579 w583] -> w570
              tunnel: [w576 w578 w582] -> w569
              tunnel: w568 -> [w575 w579 w598]
              tunnel: w567 -> [w576 w580 w599]
              tunnel: w564 -> [_ _ w589]
              tunnel: w565 -> [_ _ _]
              frame "En mouvement...", Default {
              }
              frame "Stopée" {
                n232 = Bundle By Name(cluster=w580, "Status Platine"=Status_Platine."Veille") -> (w578:refnum<class "UI SmarAct.lvclass">)
              }
              frame "Veille" {
                n233 = call "Scanner.vi"("Inc:(um)"=w589, "error in (no error)"=w598, "UI SA en entrée"=w599) -> ("error out"=w594:errorcluster, "Nbre de scans"=w600:i32, "UI SA en sortie"=w596:refnum<class "UI SmarAct.lvclass">)  [unwired: 6 in]
                n234 = Unbundle By Name(w596) -> ("Début (um)"=w595:i32, "Autocco Value"=w591:dbl[])
                n235 = call "Stall Data Flow.vim"("value in"=w594, "milliseconds to wait"=u32 200) -> ("value out"=w593:errorcluster)  [unwired: 1 out]
                n236 = for {
                  N: w600 -> [_]
                  shift-right: [w624] -> w587
                  shift-left: w593 -> [w612]
                  tunnel: w596 -> [w613]
                  tunnel: [w615] -> w597
                  tunnel: w595 -> [w618]
                  tunnel: [w621] -> w590
                  shift-right: [w601] -> _
                  shift-left: w591 -> [w622]
                  tunnel: w589 -> [w619]
                  i -> [w620]
                  stop <- "Stop Scan" stop-if-true
                  n237 = local read "PosX.Curs-0"() -> (w616:dbl)
                  n238 = local read "PosX.Curs-1"() -> (w617:dbl)
                  n239 = call "Scan For Loop.vi"("UI SA en entrée"=w613, "itération"=w620, "Inc:(um)"=w619, "PosX.Curs-1"=w617, "Début (um)"=w618, "error in (no error)"=w612, "PosX.Curs-0"=w616) -> ("Nbr de Scans"=→"scan en cours(N)":i32, "UI SA en sortie"=w609:refnum<class "UI SmarAct.lvclass">, "Aire"=w602:dbl, "Spectrogramme One Acq"=w615:dbl[][], "error out"=w611:errorcluster)  [unwired: 4 in]
                  "FROG Trace" <- w615
                  n240 = Build Array (concatenate)(w622, w602) -> (w601:dbl[])
                  n241 = local write "Aire"(w602) -> ()
                  n242 = call "Fit Gaussien.vi"("error in (no error)"=w611, "Signal Autocco"=w601, "UI SA en entrée"=w609) -> ("error out"=w610:errorcluster, "Best Gaussian Fit"=w606:dbl[], "Signal Autocco Norm"=w607:dbl[], "UI SA en sortie"=w608:refnum<class "UI SmarAct.lvclass">, "FWHM(Gauss)"=→"FWHM(Gauss)":dbl, "FWHM(Sech2)"=→"FWHM(Sech2)":dbl)  [unwired: 3 in]
                  n243 = Bundle By Name(cluster=w608, "Autocco Value"=w601) -> (w621:refnum<class "UI SmarAct.lvclass">)
                  n244 = Build Array(w607, w606) -> (→"Autoccorrélation":dbl[][])
                  n245 = call "Stall Data Flow.vim"("value in"=w610, "milliseconds to wait"=u32 100 ("n millisecondes")) -> ("value out"=w624:errorcluster)  [unwired: 1 out]
                }
                n246 = Bundle By Name(cluster=w590, "FROG Trace"=w597) -> (w588:refnum<class "UI SmarAct.lvclass">)
                n247 = call "Stall Data Flow.vim"("value in"=w587, "milliseconds to wait"=u32 1000) -> ("value out"=w586:errorcluster)  [unwired: 1 out]
                n248 = call "GoToPosAbs.vi"("error in (no error)"=w586, "UI SA en entrée"=w588) -> ("error out"=w584:errorcluster, "UI SA en sortie"=w581:refnum<class "UI SmarAct.lvclass">)  [unwired: 8 in]
                n249 = call "rql_Start Acquisition.vi"("error in"=w584, "UI SmarAct in"=w581) -> ("error out"=w583:errorcluster, "dup UI SmarAct out"=w582:refnum<class "UI SmarAct.lvclass">)  [unwired: 8 in]
              }
            }
          }
          frame "Update début scan" {
            # "update la valeur du début du scan"
            n250 = Variant To Data(error in=w639, type=T28 {"Début (um)"=0} ("Data"), Variant=w637) -> (data=w636:T28, error out=w635:errorcluster)
            n251 = Unbundle By Name(w636) -> ("Début (um)"=w630:i32)
            n252 = Bundle By Name(cluster=w632, "Début (um)"=w630) -> (w631:refnum<class "UI SmarAct.lvclass">)
            n253 = To Double Precision Float(number=w630) -> (double precision float=w634:dbl)
            n254 = call "Conversion umToFs.vi"("error in (no error)"=w635, "um"=w634, "UI SA en entrée"=w631) -> ("error out"=w629:errorcluster, "Fs"=→"fs2":ext, "UI SA en sortie"=w627:refnum<class "UI SmarAct.lvclass">)  [unwired: 6 in]
            n255 = call "rql_Write init file.vi"("error in"=w629, "UI SmarAct in"=w627) -> ("error out"=w628:errorcluster, "dup UI SmarAct out"=w626:refnum<class "UI SmarAct.lvclass">)  [unwired: 8 in]
          }
          frame "Update fin scan" {
            # "Update la valeur de fin du scan"
            n256 = Variant To Data(error in=w652, type=T29 {"fin (um)"=0} ("Data"), Variant=w650) -> (data=w649:T29, error out=w644:errorcluster)
            n257 = Unbundle By Name(w649) -> ("fin (um)"=w641:i32)
            n258 = Bundle By Name(cluster=w653, "fin (um)"=w641) -> (w647:refnum<class "UI SmarAct.lvclass">)
            n259 = To Double Precision Float(number=w641) -> (double precision float=w648:dbl)
            n260 = call "Conversion umToFs.vi"("error in (no error)"=w644, "um"=w648, "UI SA en entrée"=w647) -> ("error out"=w643:errorcluster, "Fs"=→"fs 3":ext, "UI SA en sortie"=w646:refnum<class "UI SmarAct.lvclass">)  [unwired: 6 in]
            n261 = call "rql_Write init file.vi"("error in"=w643, "UI SmarAct in"=w646) -> ("error out"=w642:errorcluster, "dup UI SmarAct out"=w645:refnum<class "UI SmarAct.lvclass">)  [unwired: 8 in]
          }
          frame "Save Spectrogramme" {
            # "Sauvegarde le spectrogramme"
            n262 = Variant To Data(error in=w672, type=T32 {"Save"=FALSE} ("Data"), Variant=w670) -> (data=w669:T32, error out=w667:errorcluster)
            n263 = Unbundle By Name(w660) -> ("N"=w659:i32, "FROG Trace"=w658:dbl[][], "Nbre de scans"=w657:i32, "WL Values"=w656:dbl[], "Inc:(um)"=w654:dbl)
            n264 = local read "Transposer Le spectrogramme"() -> (w655:bool)
            n265 = Unbundle By Name(w669) -> ("Save"=w661:bool)
            n266 = To Double Precision Float(number=w654) -> (double precision float=w662:dbl)
            n267 = Bundle By Name(cluster=T30 {"Save SpecTG"=FALSE, "Paramètres longueur d'onde"={"N"=2068, "lambda_0"=200.6310762, "lambda_c"=674.8888701568728, "d_lambda"=0.44435503366880597}, "FROG Trace"=[], "pas (um)"=0.0, "Nbre de scans"=0, "WL Values"=[], "Transposer L'image"=FALSE} ("Data in"), "Transposer L'image"=w655, "Paramètres longueur d'onde.N"=w659, "FROG Trace"=w658, "Nbre de scans"=w657, "WL Values"=w656, "pas (um)"=w662, "Save SpecTG"=w661) -> (w665:T30)
            n268 = Unbundle By Name(w660) -> ("File mainpulate"=w663:refnum<class "File manipulate.lvclass">)
            n269 = call "rqp_Save Spectrogramme Data.vi"("Caller in"=w660, "error in"=w667, "Data in"=w665, "File manipulate in"=w663) -> ("error out"=w666:errorcluster, "dup Caller out"=w664:refnum<class "UI SmarAct.lvclass">)  [unwired: 5 in, 1 out]
          }
          frame "Update Pas Platine" {
            # "Mise à jour des pas de la platine"
            n270 = Variant To Data(error in=w682, type=T33 {"Inc:(um)"=0.0} ("Data"), Variant=w680) -> (data=w679:T33, error out=w678:errorcluster)
            n271 = Unbundle By Name(w679) -> ("Inc:(um)"=w673:dbl)
            n272 = Bundle By Name(cluster=w676, "Inc:(um)"=w673) -> (w674:refnum<class "UI SmarAct.lvclass">)
            n273 = call "rql_Write init file.vi"("error in"=w678, "UI SmarAct in"=w674) -> ("error out"=w677:errorcluster, "dup UI SmarAct out"=w675:refnum<class "UI SmarAct.lvclass">)  [unwired: 8 in]
          }
          frame "Switch Platine" {
            # "You can delete this warning once\nyou add code to this MHL case"
            # "Switch entre les platine smaract et newport"
            n274 = Variant To Data(error in=w696, type=T34 {"Platine Switch"=FALSE} ("Data"), Variant=w693) -> (data=w692:T34, error out=w695:errorcluster)
            n275 = Unbundle By Name(w692) -> ("Platine Switch"=w690:bool)
            n276 = Bundle By Name(cluster=w697, "Platine Switch"=w690) -> (w684:refnum<class "UI SmarAct.lvclass">)
            n277 = xnode ("Error_Ring")() -> ("sortie d'erreur"=w691:errorcluster)
            n278 = Merge Errors(w695, w691) -> (w686:errorcluster)
            n279 = call "Initier attributs.vi"("error in (no error)"=w686, "Main/Refresh"="Refresh", "UI SA en entrée"=w684) -> ("error out"=w685:errorcluster, "UI SA en sortie"=w683:refnum<class "UI SmarAct.lvclass">)  [unwired: 7 in]
            n280 = call "rql_Write init file.vi"("error in"=w685, "UI SmarAct in"=w683) -> ("error out"=w689:errorcluster, "dup UI SmarAct out"=w688:refnum<class "UI SmarAct.lvclass">)  [unwired: 8 in]
          }
          frame "Update Port COM" {
            # "mise à jour du port com de la platine newport"
            n281 = Variant To Data(error in=w710, type=T35 {"Port COM"=""} ("Data"), Variant=w708) -> (data=w707:T35, error out=w703:errorcluster)
            n282 = Unbundle By Name(w707) -> ("Port COM"=w706:refnum<visa-resource-name>)
            n283 = Bundle By Name(cluster=w711, "Port COM"=w706) -> (w701:refnum<class "UI SmarAct.lvclass">)
            n284 = call "Init SMC100.vi"("error in (no error)"=w703, "UI SA en entrée"=w701) -> ("error out"=w702:errorcluster, "ControllerVersion"=w699:string, "UI SA en sortie"=w700:refnum<class "UI SmarAct.lvclass">)  [unwired: 6 in, 1 out]
            n285 = local write "Version Controller"(w699) -> ()
            n286 = call "rql_Write init file.vi"("error in"=w702, "UI SmarAct in"=w700) -> ("error out"=w705:errorcluster, "dup UI SmarAct out"=w704:refnum<class "UI SmarAct.lvclass">)  [unwired: 8 in]
          }
          frame "Update Calib" {
            # "Mise à jour de la calibration"
            n287 = Variant To Data(error in=w728, type=T37 {"Calib?"=FALSE} ("Data"), Variant=w725) -> (data=w724:T37, error out=w727:errorcluster)
            n288 = Unbundle By Name(w724) -> ("Calib?"=w712:bool)
            n289 = xnode ("Error_Ring")() -> ("sortie d'erreur"=w723:errorcluster)
            n290 = Bundle By Name(cluster=w718, "Calib?"=w712) -> (w713:refnum<class "UI SmarAct.lvclass">)
            n291 = Merge Errors(w727, w723) -> (w720:errorcluster)
            n292 = Unbundle By Name(w713) -> ("Spectro Acq"=w719:refnum<class "Spectro Acquisition.lvclass">)
            n293 = Bundle By Name(cluster=T36 {"Calib?"=FALSE} ("Data"), "Calib?"=w712) -> (w721:T36)
            n294 = call "rqp_Appliquer calibration.vi"("Caller in"=w713, "error in"=w720, "Data in"=w721, "Spectro Acquisition in"=w719) -> ("error out"=w717:errorcluster, "dup Caller out"=w715:refnum<class "UI SmarAct.lvclass">)  [unwired: 5 in, 1 out]
            n295 = call "rql_Write init file.vi"("error in"=w717, "UI SmarAct in"=w715) -> ("error out"=w716:errorcluster, "dup UI SmarAct out"=w714:refnum<class "UI SmarAct.lvclass">)  [unwired: 8 in]
          }
          frame "Update Incr Scan" {
            # "You can delete this warning once\nyou add code to this MHL case"
            # "Mise à jour de la valeur d'incrémentation du scan"
            n296 = Variant To Data(error in=w740, type=T38 {"Inc Scan:(um)"=0.0} ("Data"), Variant=w737) -> (data=w736:T38, error out=w739:errorcluster)
            n297 = Unbundle By Name(w736) -> ("Inc Scan:(um)"=w734:dbl)
            n298 = xnode ("Error_Ring")() -> ("sortie d'erreur"=w735:errorcluster)
            n299 = Bundle By Name(cluster=w741, "Inc Scan:(um)"=w734) -> (w733:refnum<class "UI SmarAct.lvclass">)
            n300 = Merge Errors(w739, w735) -> (w731:errorcluster)
            n301 = call "rql_Write init file.vi"("error in"=w731, "UI SmarAct in"=w733) -> ("error out"=w730:errorcluster, "dup UI SmarAct out"=w732:refnum<class "UI SmarAct.lvclass">)  [unwired: 8 in]
          }
          frame "Update Controller Adress SMC100" {
            # "Update l'adresse du controleur SMC 100"
            n302 = Variant To Data(error in=w753, type=T39 {"Adresse SMC100"=0} ("Data"), Variant=w750) -> (data=w749:T39, error out=w752:errorcluster)
            n303 = Unbundle By Name(w749) -> ("Adresse SMC100"=w747:i32)
            n304 = Bundle By Name(cluster=w754, "Adresse SMC100"=w747) -> (w744:refnum<class "UI SmarAct.lvclass">)
            n305 = xnode ("Error_Ring")() -> ("sortie d'erreur"=w748:errorcluster)
            n306 = Merge Errors(w752, w748) -> (w746:errorcluster)
            n307 = call "rql_Write init file.vi"("error in"=w746, "UI SmarAct in"=w744) -> ("error out"=w745:errorcluster, "dup UI SmarAct out"=w743:refnum<class "UI SmarAct.lvclass">)  [unwired: 8 in]
          }
        }
        n308 = call-dynamic "Error Handler.vi"("Worker"=w118, "error_in"=w120) -> ("error out"=w123:errorcluster, "Stop Loop"=w116:bool, "Worker out"=w122:refnum<class "UI SmarAct.lvclass">)  [unwired: 7 in]
      }
      n309 = call-dynamic "Setup EHL.vi"("Worker"=w107) -> ("Worker out"=w108:refnum<class "UI SmarAct.lvclass">)  [unwired: 14 in]
      n310 = while "Event Handling Loop" {
        shift-right: [w764] -> w111
        shift-left: w112 -> [w763]
        tunnel: [w759] -> w109
        tunnel: errorcluster {"status"=FALSE, "code"=0, "source"=""} ("error constant") -> [w761]
        shift-right: [w757] -> _
        shift-left: w108 -> [w762]
        stop <- w756 stop-if-true
        # "Event Handling Loop"
        n311 = event shown="[29] \"Adresse SMC100\": Valeur changée" {
          selector: w763 -> [_ _ _ _ _ _ _ _ _ _ _ _ _ _ _ _ _ _ _ _ _ _ _ _ _ _ _ _ _ _]
          dyn-events: [_ _ _ _ _ _ _ _ _ _ _ _ _ _ _ _ _ _ _ _ _ _ _ _ _ _ _ _ _ _] -> w764
          timeout: _ -> [_ _ _ _ _ _ _ _ _ _ _ _ _ _ _ _ _ _ _ _ _ _ _ _ _ _ _ _ _ _]
          tunnel: [w768 w775 w783 w787 w794 w798 w802 w806 w810 w814 w821 w828 w835 w840 w847 w853 w857 w864 w868 w873 w878 w886 w892 w897 w904 w911 w913 w925 w932 w937] -> w760
          tunnel: w761 -> [w769 w771 w784 w788 w795 w799 w803 w807 w811 w815 w822 w829 w836 w841 w848 w854 w858 w865 w869 w874 w879 w887 w893 w898 w905 w912 w915 w926 w933 w938]
          tunnel: w762 -> [w767 w770 w782 w786 w793 w797 w801 w805 w809 w813 w820 w827 w834 w839 w845 w852 w856 w860 w867 w871 w876 w881 w889 w896 w903 w907 w917 w924 w931 w940]
          tunnel: [w766 w774 w781 w785 w792 w796 w800 w804 w808 w812 w819 w826 w833 w838 w846 w851 w855 w859 w866 w872 w877 w885 w888 w895 w902 w906 w916 w923 w930 w939] -> w758
          event User Event {
            # "This case and its contents must always be included in every EHL that you use, so that the framework can automatically stop the EHL."
            # "EHL Stop Event. This EHL exits from this case."
            n312 = event-data() -> ("Stop Event Data"=w765:variant)  [unwired: 1 in]
            n313 = call-dynamic "EHL Stop - EHL Case.vi"("error in"=w769, "Stop Event Data"=w765, "Worker"=w767) -> ("error out"=w768:errorcluster, "Worker out"=w766:refnum<class "UI SmarAct.lvclass">)  [unwired: 7 in]
          }
          event Panel Close? {
            # "Use this VI when you want to exit this Worker. This VI will call the Start Exiting case of this Worker. This is the correct way to exit your Worker."
            # "Calls the Start Exiting case of this Worker. This will start the exiting sequence of this Worker."
            n314 = event-data() -> ()  [unwired: 1 in, 1 out]
            n315 = property class="UI SA"(reference=w770) -> (reference out=w773:refnum<class "UI SmarAct.lvclass">, "Accessors:Read:Public API:Queue"=w772:refnum<class "Message Queue.lvclass">)  [unwired: 1 in, 1 out]
            n316 = call-dynamic "Worker Start Exiting.vi"("error_in"=w771, "Message Queue"=w772, "Worker"=w773) -> ("error out"=w775:errorcluster, "dup Worker out"=w774:refnum<class "UI SmarAct.lvclass">)  [unwired: 7 in]
            n317 = event-data ("Nœud de filtre d'événements")("Discard?"=TRUE) -> ()  [unwired: 1 in, 1 out]
          }
          event "Connecter": Value Change {
            n318 = event-data() -> ("NewVal"=w777:bool)  [unwired: 1 in, 1 out]
            n319 = Bundle By Name ("Assembler par nom")(cluster=T7 {"String"="", "Connect?"=FALSE} ("Data"), "Connect?"=w777) -> (w779:T7)
            n320 = call "rql_Connect MCS.vi"("Show in Debugger?"=TRUE, "error in"=w784, "Data in"=w779, "UI SmarAct in"=w782) -> ("error out"=w783:errorcluster, "dup UI SmarAct out"=w781:refnum<class "UI SmarAct.lvclass">)  [unwired: 6 in]
          }
          event "Refresh": Value Change {
            n321 = event-data() -> ()  [unwired: 1 in, 1 out]
            n322 = call "rql_Refresh.vi"("error in"=w788, "UI SmarAct in"=w786) -> ("error out"=w787:errorcluster, "dup UI SmarAct out"=w785:refnum<class "UI SmarAct.lvclass">)  [unwired: 8 in]
          }
          event "Channel": Value Change {
            n323 = event-data() -> ("NewVal"=w789:u32)  [unwired: 1 in]
            n324 = Bundle By Name ("Assembler par nom")(cluster=T10 {"Channel"=0} ("Data"), "Channel"=w789) -> (w790:T10)
            n325 = call "rql_Update channel.vi"("error in"=w795, "Data in"=w790, "UI SmarAct in"=w793) -> ("error out"=w794:errorcluster, "dup UI SmarAct out"=w792:refnum<class "UI SmarAct.lvclass">)  [unwired: 7 in]
          }
          event "get position": Value Change {
            n326 = event-data() -> ()  [unwired: 1 in, 1 out]
            n327 = call "rql_Get position.vi"("error in"=w799, "UI SmarAct in"=w797) -> ("error out"=w798:errorcluster, "dup UI SmarAct out"=w796:refnum<class "UI SmarAct.lvclass">)  [unwired: 8 in]
          }
          event "Find Zero": Value Change {
            n328 = event-data() -> ()  [unwired: 1 in, 1 out]
            n329 = call "rql_Find Reference Zero.vi"("error in"=w803, "UI SmarAct in"=w801) -> ("error out"=w802:errorcluster, "dup UI SmarAct out"=w800:refnum<class "UI SmarAct.lvclass">)  [unwired: 8 in]
          }
          event "Set Zero": Value Change {
            n330 = event-data() -> ()  [unwired: 1 in, 1 out]
            n331 = call "rql_Set Zero Position.vi"("error in"=w807, "UI SmarAct in"=w805) -> ("error out"=w806:errorcluster, "dup UI SmarAct out"=w804:refnum<class "UI SmarAct.lvclass">)  [unwired: 8 in]
          }
          event "Forward CL": Value Change {
            n332 = event-data() -> ()  [unwired: 1 in, 1 out]
            n333 = call "rql_Forward CloseLoop.vi"("error in"=w811, "UI SmarAct in"=w809) -> ("error out"=w810:errorcluster, "dup UI SmarAct out"=w808:refnum<class "UI SmarAct.lvclass">)  [unwired: 8 in]
          }
          event "Back CL": Value Change {
            n334 = event-data() -> ()  [unwired: 1 in, 1 out]
            n335 = call "rql_Back Closed Loog.vi"("error in"=w815, "UI SmarAct in"=w813) -> ("error out"=w814:errorcluster, "dup UI SmarAct out"=w812:refnum<class "UI SmarAct.lvclass">)  [unwired: 8 in]
          }
          event "max freq (50 ... 18 500)": Value Change {
            n336 = event-data() -> ("NewVal"=w817:u32)  [unwired: 1 in]
            n337 = Bundle By Name ("Assembler par nom")(cluster=T17 {"max freq (50 ... 18 500)"=200} ("Data"), "max freq (50 ... 18 500)"=w817) -> (w816:T17)
            n338 = call "rql_Update Fréquence.vi"("error in"=w822, "Data in"=w816, "UI SmarAct in"=w820) -> ("error out"=w821:errorcluster, "dup UI SmarAct out"=w819:refnum<class "UI SmarAct.lvclass">)  [unwired: 7 in]
          }
          event "speed (0 ... 100 000 000)": Value Change {
            n339 = event-data() -> ("NewVal"=w823:u32)  [unwired: 1 in]
            n340 = Bundle By Name ("Assembler par nom")(cluster=T18 {"speed (0 ... 100 000 000)"=1000000} ("Data"), "speed (0 ... 100 000 000)"=w823) -> (w824:T18)
            n341 = call "rql_Update Vitesse.vi"("error in"=w829, "Data in"=w824, "UI SmarAct in"=w827) -> ("error out"=w828:errorcluster, "dup UI SmarAct out"=w826:refnum<class "UI SmarAct.lvclass">)  [unwired: 7 in]
          }
          event "Abs/Rel": Value Change {
            n342 = event-data() -> ("NewVal"=w831:bool)  [unwired: 1 in]
            n343 = Bundle By Name ("Assembler par nom")(cluster=T19 {"Abs/Rel"=FALSE} ("Data"), "Abs/Rel"=w831) -> (w830:T19)
            n344 = call "rql_Mode déplacement.vi"("error in"=w836, "Data in"=w830, "UI SmarAct in"=w834) -> ("error out"=w835:errorcluster, "dup UI SmarAct out"=w833:refnum<class "UI SmarAct.lvclass">)  [unwired: 7 in]
          }
          event "Platine Switch": Value Change {
            n345 = event-data() -> ("NewVal"=w843:bool)  [unwired: 1 in]
            n346 = Bundle By Name ("Assembler par nom")(cluster=T34 {"Platine Switch"=FALSE} ("Data"), "Platine Switch"=w843) -> (w837:T34)
            n347 = call "rql_Switch Platine.vi"("error in"=w841, "Data in"=w837, "UI SmarAct in"=w839) -> ("error out"=w840:errorcluster, "dup UI SmarAct out"=w838:refnum<class "UI SmarAct.lvclass">)  [unwired: 7 in]
          }
          event "Port COM": Value Change {
            n348 = event-data() -> ("NewVal"=w850:refnum<visa-resource-name>)  [unwired: 1 in]
            n349 = Bundle By Name ("Assembler par nom")(cluster=T35 {"Port COM"=""} ("Data"), "Port COM"=w850) -> (w844:T35)
            n350 = call "rql_Update Port COM.vi"("error in"=w848, "Data in"=w844, "UI SmarAct in"=w845) -> ("error out"=w847:errorcluster, "dup UI SmarAct out"=w846:refnum<class "UI SmarAct.lvclass">)  [unwired: 7 in]
          }
          event "Connecter Spectro": Value Change {
            n351 = event-data() -> ()  [unwired: 1 in, 1 out]
            n352 = call "rql_Initialise Spectromètre.vi"("error in"=w854, "UI SmarAct in"=w852) -> ("error out"=w853:errorcluster, "dup UI SmarAct out"=w851:refnum<class "UI SmarAct.lvclass">)  [unwired: 8 in]
          }
          event "Stop moteur": Value Change {
            n353 = event-data() -> ()  [unwired: 1 in, 1 out]
            n354 = call "rql_Stop platine.vi"("error in"=w858, "UI SmarAct in"=w856) -> ("error out"=w857:errorcluster, "dup UI SmarAct out"=w855:refnum<class "UI SmarAct.lvclass">)  [unwired: 8 in]
          }
          event "Tps Int.(ms)": Value Change {
            n355 = event-data() -> ("NewVal"=w862:u32)  [unwired: 1 in]
            n356 = Bundle By Name ("Assembler par nom")(cluster=T24 {"Tps Int.(ms)"=0} ("Data"), "Tps Int.(ms)"=w862) -> (w861:T24)
            n357 = call "rql_Update Tps Int.vi"("error in"=w865, "Data in"=w861, "UI SmarAct in"=w860) -> ("error out"=w864:errorcluster, "dup UI SmarAct out"=w859:refnum<class "UI SmarAct.lvclass">)  [unwired: 7 in]
          }
          event "Start Acquisition": Value Change {
            n358 = event-data() -> ()  [unwired: 1 in, 1 out]
            n359 = call "rql_Start Acquisition.vi"("error in"=w869, "UI SmarAct in"=w867) -> ("error out"=w868:errorcluster, "dup UI SmarAct out"=w866:refnum<class "UI SmarAct.lvclass">)  [unwired: 8 in]
          }
          event "Stop Acquisition": Value Change {
            n360 = event-data() -> ()  [unwired: 1 in, 1 out]
            n361 = Unbundle By Name(w871) -> ("Spectro Acq"=w870:refnum<class "Spectro Acquisition.lvclass">)
            n362 = call "rqp_Stop Acquisition.vi"("Caller in"=w871, "error in"=w874, "Spectro Acquisition in"=w870) -> ("error out"=w873:errorcluster, "dup Caller out"=w872:refnum<class "UI SmarAct.lvclass">)  [unwired: 6 in, 1 out]
          }
          event "BKG": Value Change {
            n363 = event-data() -> ()  [unwired: 1 in, 1 out]
            n364 = Unbundle By Name(w876) -> ("Spectro Acq"=w875:refnum<class "Spectro Acquisition.lvclass">)
            n365 = call "rqp_Update Background.vi"("Caller in"=w876, "error in"=w879, "Spectro Acquisition in"=w875) -> ("error out"=w878:errorcluster, "dup Caller out"=w877:refnum<class "UI SmarAct.lvclass">)  [unwired: 6 in, 1 out]
          }
          event "BKG?": Value Change {
            n366 = event-data() -> ("NewVal"=w882:bool)  [unwired: 1 in]
            n367 = Unbundle By Name(w881) -> ("Spectro Acq"=w880:refnum<class "Spectro Acquisition.lvclass">)
            n368 = Bundle By Name(cluster=T40 {"BackGround?"=FALSE} ("Data in"), "BackGround?"=w882) -> (w883:T40)
            n369 = call "rqp_Appliquer BKG.vi"("Caller in"=w881, "error in"=w887, "Data in"=w883, "Spectro Acquisition in"=w880) -> ("error out"=w886:errorcluster, "dup Caller out"=w885:refnum<class "UI SmarAct.lvclass">)  [unwired: 5 in, 1 out]
          }
          event "Calib?": Value Change {
            n370 = event-data() -> ("NewVal"=w894:bool)  [unwired: 1 in]
            n371 = Bundle By Name(cluster=T37 {"Calib?"=FALSE} ("Data"), "Calib?"=w894) -> (w890:T37)
            n372 = call "rql_Update Calib.vi"("error in"=w893, "Data in"=w890, "UI SmarAct in"=w889) -> ("error out"=w892:errorcluster, "dup UI SmarAct out"=w888:refnum<class "UI SmarAct.lvclass">)  [unwired: 7 in]
          }
          event "Start Scan": Value Change {
            n373 = event-data() -> ()  [unwired: 1 in, 1 out]
            n374 = call "rql_Start Scan.vi"("error in"=w898, "UI SmarAct in"=w896) -> ("error out"=w897:errorcluster, "dup UI SmarAct out"=w895:refnum<class "UI SmarAct.lvclass">)  [unwired: 8 in]
          }
          event "Début (um)": Value Change {
            n375 = event-data() -> ("NewVal"=w900:i32)  [unwired: 1 in]
            n376 = Bundle By Name(cluster=T28 {"Début (um)"=0} ("Data"), "Début (um)"=w900) -> (w899:T28)
            n377 = call "rql_Update début scan.vi"("error in"=w905, "Data in"=w899, "UI SmarAct in"=w903) -> ("error out"=w904:errorcluster, "dup UI SmarAct out"=w902:refnum<class "UI SmarAct.lvclass">)  [unwired: 7 in]
          }
          event "Inc Scan:(um)": Value Change {
            n378 = event-data() -> ("NewVal"=w909:dbl)  [unwired: 1 in]
            n379 = Bundle By Name(cluster=T38 {"Inc Scan:(um)"=0.0} ("Data"), "Inc Scan:(um)"=w909) -> (w908:T38)
            n380 = call "rql_Update Incr Scan.vi"("error in"=w912, "Data in"=w908, "UI SmarAct in"=w907) -> ("error out"=w911:errorcluster, "dup UI SmarAct out"=w906:refnum<class "UI SmarAct.lvclass">)  [unwired: 7 in]
          }
          event "fin (um)": Value Change {
            n381 = event-data() -> ("NewVal"=w918:i32)  [unwired: 1 in]
            n382 = Bundle By Name(cluster=T29 {"fin (um)"=0} ("Data"), "fin (um)"=w918) -> (w914:T29)
            n383 = call "rql_Update fin scan.vi"("error in"=w915, "Data in"=w914, "UI SmarAct in"=w917) -> ("error out"=w913:errorcluster, "dup UI SmarAct out"=w916:refnum<class "UI SmarAct.lvclass">)  [unwired: 7 in]
          }
          event "Save FROG Trace": Value Change {
            n384 = event-data() -> ()  [unwired: 1 in, 1 out]
            n385 = Bundle By Name(cluster=T32 {"Save"=FALSE} ("Data"), "Save"="Save FROG Trace") -> (w921:T32)
            n386 = call "rql_Save Spectrogramme.vi"("error in"=w926, "Data in"=w921, "UI SmarAct in"=w924) -> ("error out"=w925:errorcluster, "dup UI SmarAct out"=w923:refnum<class "UI SmarAct.lvclass">)  [unwired: 7 in]
          }
          event "Inc:(um)": Value Change {
            w929 = T33 {"Inc:(um)"=0.0}  # Data in
            n387 = event-data() -> ("NewVal"=w927:dbl)  [unwired: 1 in]
            n388 = Bundle By Name(cluster=w929, "Inc:(um)"=w927) -> (w928:T33)
            n389 = call "rql_Update Pas Platine.vi"("error in"=w933, "Data in"=w928, "UI SmarAct in"=w931) -> ("error out"=w932:errorcluster, "dup UI SmarAct out"=w930:refnum<class "UI SmarAct.lvclass">)  [unwired: 7 in]
          }
          event "Adresse SMC100": Value Change {
            n390 = event-data() -> ("NewVal"=w934:i32)  [unwired: 1 in]
            n391 = Bundle By Name(cluster=T39 {"Adresse SMC100"=0} ("Data"), "Adresse SMC100"=w934) -> (w935:T39)
            n392 = call "rql_Update Controller Adress SMC100.vi"("error in"=w938, "Data in"=w935, "UI SmarAct in"=w940) -> ("error out"=w937:errorcluster, "dup UI SmarAct out"=w939:refnum<class "UI SmarAct.lvclass">)  [unwired: 7 in]
          }
        }
        n393 = call-dynamic "Error Handler.vi"("Worker"=w758, "error_in"=w760) -> ("error out"=w759:errorcluster, "Stop Loop"=w756:bool, "Worker out"=w757:refnum<class "UI SmarAct.lvclass">)  [unwired: 7 in]
      }
    }
    frame Error {
      n394 = call-dynamic "Error Handler.vi"("Worker"=w942, "error_in"=w945) -> ("error out"=w943:errorcluster, "Worker out"=w941:refnum<class "UI SmarAct.lvclass">)  [unwired: 7 in, 1 out]
    }
  }
  n395 = while {
    tunnel: w3 -> [w956]
    shift-right: [w951] -> _
    shift-left: w4 -> [w955]
    stop <- w946 stop-if-true
    # "Visu Spectre et Curseurs"
    n396 = Dequeue Element(queue=w956) -> (element=w947:T3, error out=w950:errorcluster)  [unwired: 2 in, 2 out]
    n397 = call "Calcul Aire Spectre.vi"("error in (no error)"=w950, "Data Queue"=w947, "UI SA en entrée"=w955) -> ("error out"=w946:errorcluster, "Zoom Spectre"=→"Zoom Spectre":cluster{dbl[], dbl[]}, "Spectre"=→"Spectre":T3, "UI SA en sortie"=w951:refnum<class "UI SmarAct.lvclass">, "PosX.Curs-1"=→"PosX.Curs-1":dbl, "PosX.Curs-0"=→"PosX.Curs-0":dbl, "Aire"=→"Aire":dbl)  [unwired: 2 in]
  }
  n398 = call-dynamic "Main.vi"("error in"=w36, "Spectro Acquisition in"=w10) -> ("error out"=w30:errorcluster)  [unwired: 8 in, 1 out]
  n399 = call-dynamic "Main.vi"("error in"=w36, "File manipulate in"=w9) -> ("error out"=w17:errorcluster)  [unwired: 8 in, 1 out]
  n400 = Merge Errors(w30, w17) -> (w29:errorcluster)
  n401 = property class="App"() -> ("App.Kind"=w21:T42)  [unwired: 2 in, 2 out]
  n402 = control-ref of="Ce VI"() -> (w20:refnum<vi>)
  n403 = case "Structure Condition" shown="\"Run Time System\"" w21 {
    tunnel: w20 -> [w959 _]
    tunnel: TRUE -> [w958 _]
    tunnel: FALSE -> [w957 _]
    frame "Run Time System" {
      n404 = property class="VI"(reference=w959, "TB.ShowAbortBut"=w957, "TB.ShowRunBut"=w958, "TB.ShowFreeRunBut"=w957, "TB.Visible"=w957) -> ()  [unwired: 1 in, 2 out]
    }
    frame "Development System", Default {
    }
  }
  n405 = Unregister For Events(event registration refnum=w45, error in=w46) -> (error out=w47:errorcluster)
  n406 = Merge Errors ("Fusionner les erreurs")(w47, w40, w29) -> (w44:errorcluster)
  n407 = call-dynamic "Exited Notify and Cleanup.vi"("Close FP on Exit? (T)"=FALSE, "error_in"=w44, "Worker"=w43) -> ("error out"=→"error out":errorcluster, "dup Worker out"=→"UI SmarAct out":refnum<class "UI SmarAct.lvclass">)  [unwired: 7 in]
  "Transposer Le spectrogramme" <- TRUE ("Transposer Le spectrogramme")
